vi "PSUSettingsMenu.vi"(0 "Enable":bool=TRUE, 5 "error in (no error)":errorcluster, 16 "PSU Calc":T1={"Low speed (km/s)"=2000.0, "High speed (km/s)"=3000.0, "Window (Delta-T)"=0.0, "Lower Cutoff"=0.0, "Multiplier"=0, "Low Charge (fC)"=2000.0, "High Charge (fC)"=2000.0, "High Mass (kg)"=2000.0, "Low Mass (kg)"=2000.0, "High Radius (µm) "=0.0, "Low Radius (µm)"=2000.0, "Exp. Voltage (MV)"=2000.0} {"Exp. Voltage (MV)" step=0.01 format="%#.6f"; "Window (Delta-T)" step=1.0 format="%#.0f"; "High Radius (µm)" min=0.0 max=1000.0; "High Mass (kg)" min=0.0 max=1.0; "High Charge (fC)" min=0.0 max=1000000000000.0; "High speed (km/s)" min=0.0 max=299790.0; "Low speed (km/s)" min=0.0 max=299790.0; "Low Charge (fC)" min=0.0 max=1000000000000.0; "Low Mass (kg)" min=0.0 max=1.0; "Low Radius (µm)" min=0.0 max=299792000.0; "Lower Cutoff" step=1.0 format="%#.0f"; "Multiplier" items=["1k", "10k"]}) -> (14 "Cancel 2":bool caption="Cancel", 18 "OK":bool, 19 "error out":errorcluster)   [LabVIEW 2012]
doc: "Displays a standard dialog box that prompts users to enter information, such as a user name and password.\n--------------------\n\nThis Express VI is configured as follows:\n\nMessage to Display to the User:Please Enter Experiment Settings Information For Database Storage.\nThe inputs are: \nNumber: Please Enter Group ID\nText Entry Box: Please Enter Tags:\nText Entry Box: Please Enter Experiment Description:"
uses:
  PSU Calc.ctl
  <vilib>/addons/database/Connection.llb/Conn Execute.vi
  <vilib>/addons/database/Recordset.llb/Rec Fetch Recordset Data (R).vi
  <vilib>/addons/database/Recordset.llb/Rec Destroy - Connection.vi
  PSU updated.vi
  <vilib>/addons/database/_DB Variant To Data/Database Variant To Data.xnode
  <vilib>/addons/database/NI_Database_API.lvlib
panel:
  out "Dust Density\n(kg/m^3)":dbl
  in  "Variable 2":enum32{"Velocity", "Charge", "Mass"}(radio)
  in  "Variable 1":enum32{"Velocity", "Charge", "Mass"}(radio)
  out "Lower Cutoff":dbl
  out "Window (Delta-T)":dbl
  in  "PSU update":bool caption="OK2"
  in  "Cancel":bool
  in  "OK1":bool
  # "Please Enter PSU Settings For Storage in the CCLDAS Database."
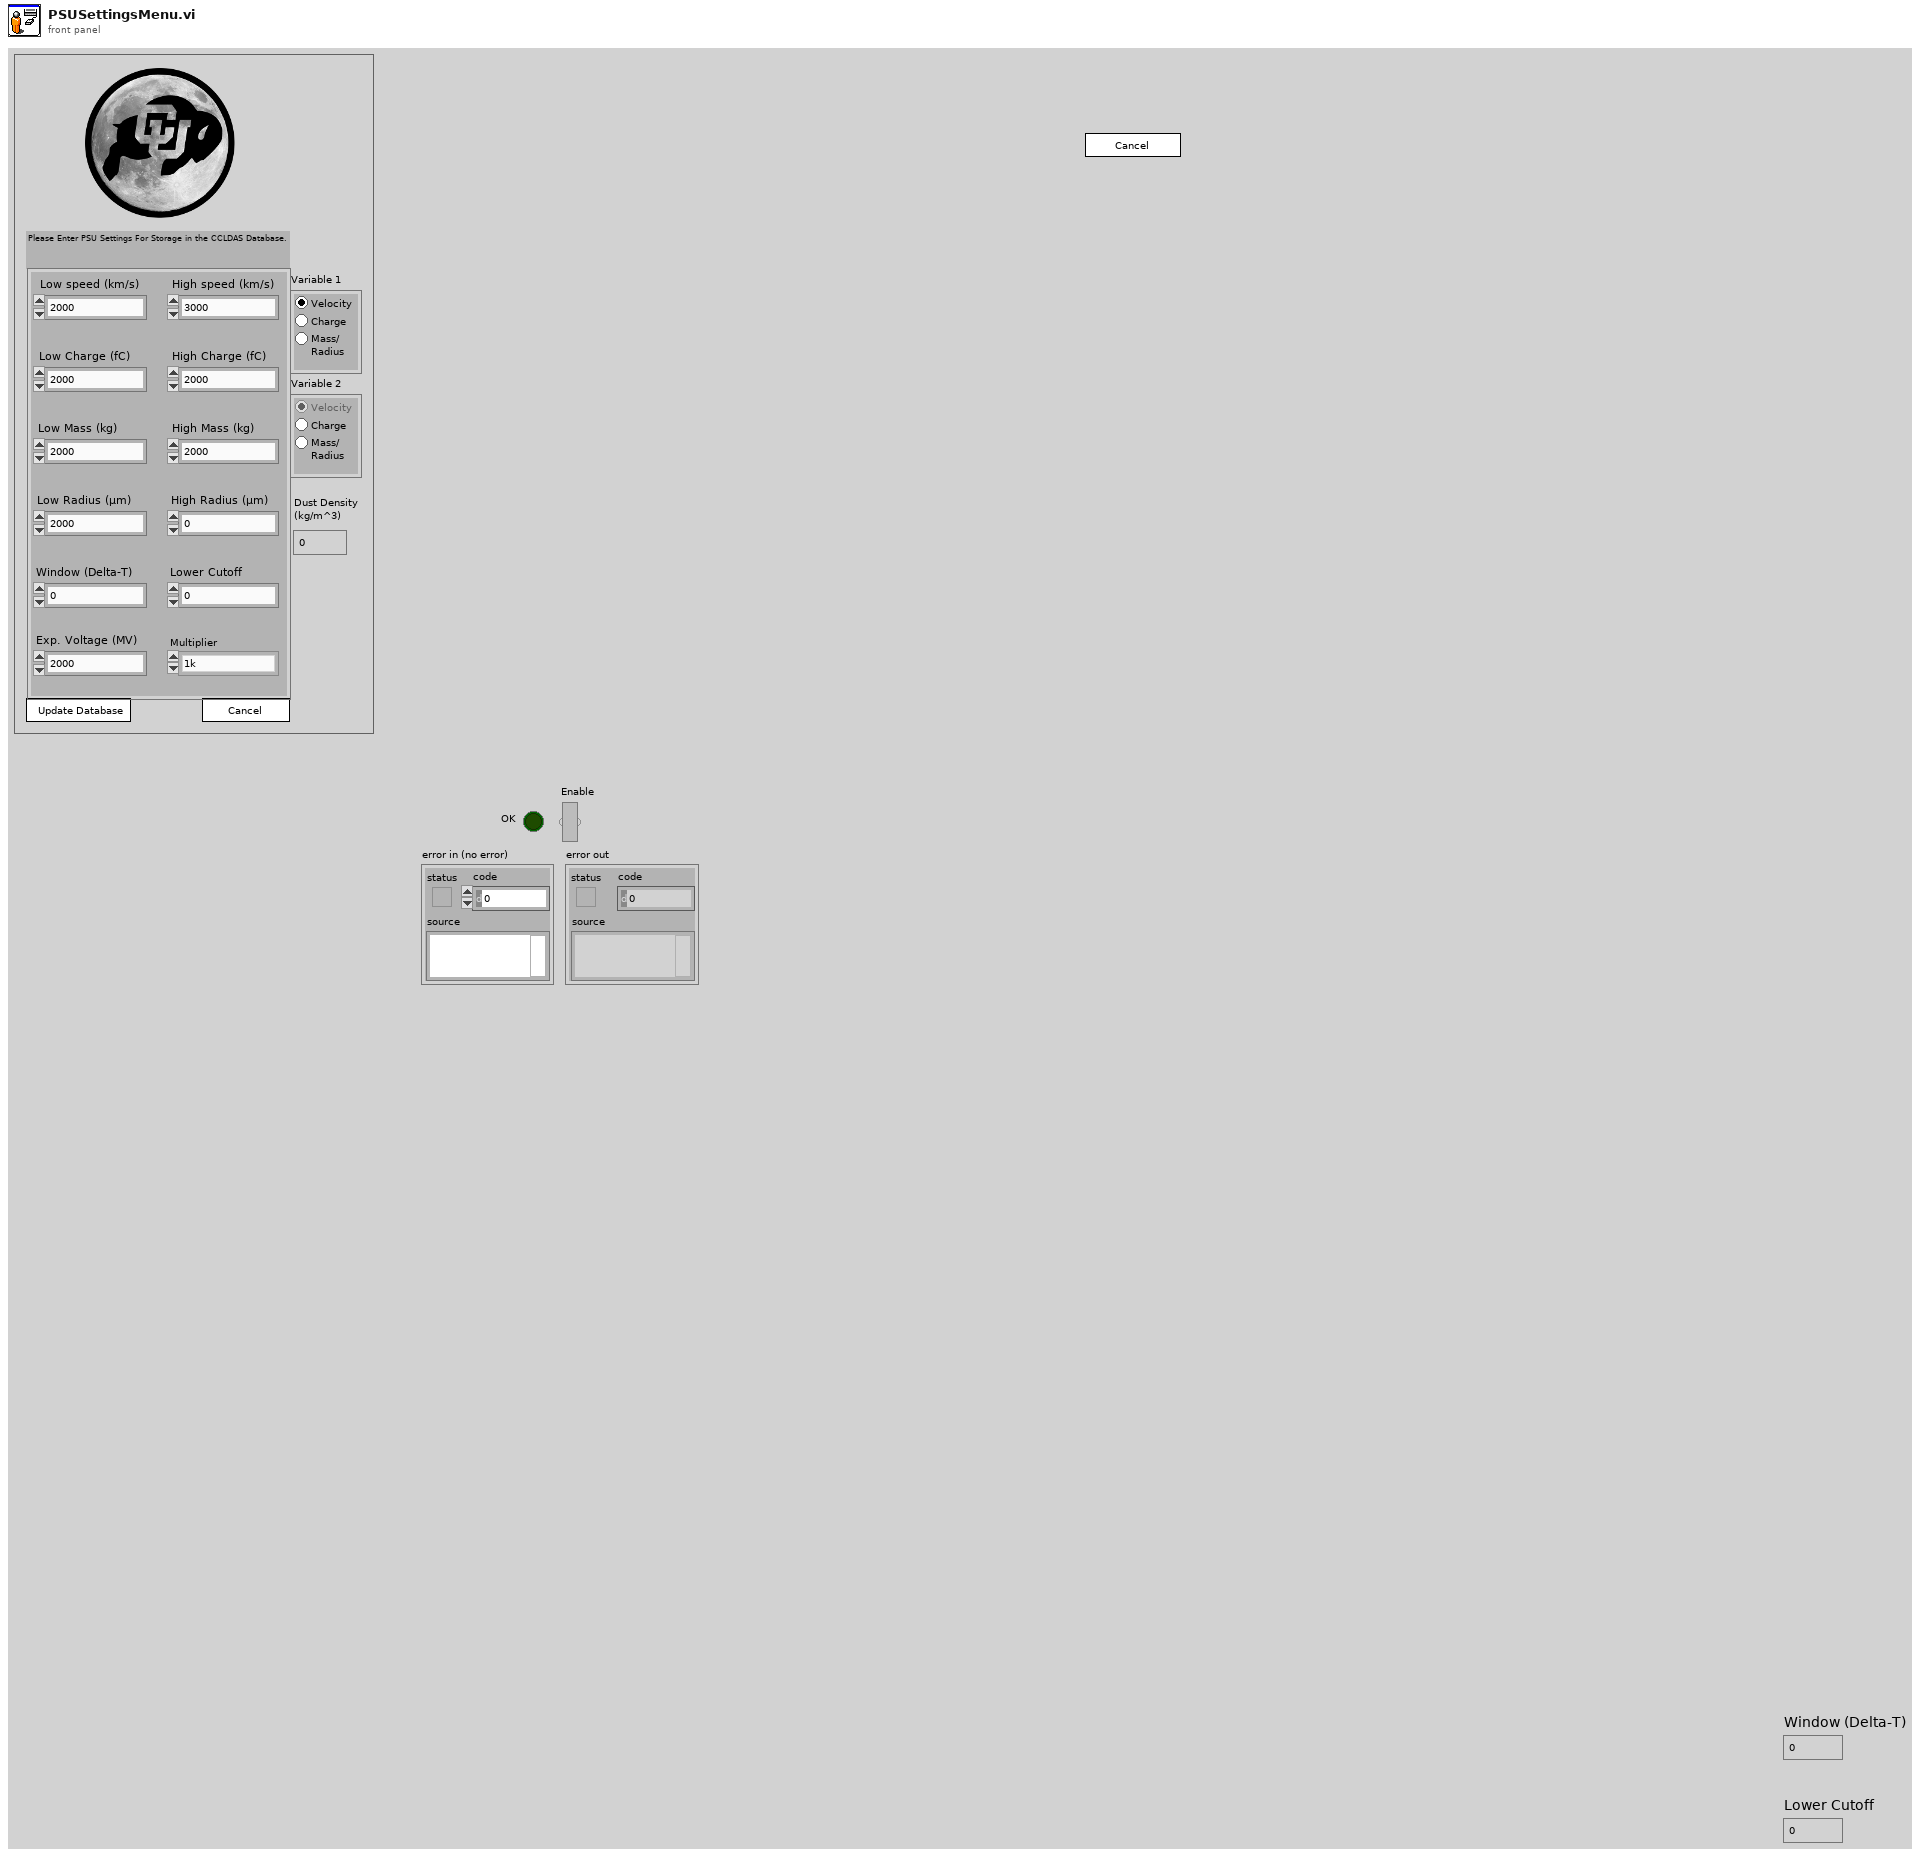
[diagram p1: front panel]
types:
  T1 = typedef "PSU Calc.ctl" = cluster{"Low speed (km/s)":dbl, "High speed (km/s)":dbl, "Window (Delta-T)":dbl, "Lower Cutoff":dbl, "Multiplier":u16, "Low Charge (fC)":dbl, "High Charge (fC)":dbl, "High Mass (kg)":dbl, "Low Mass (kg)":dbl, "High Radius (µm) ":dbl, "Low Radius (µm)":dbl, "Exp. Voltage (MV)":dbl}
  T2 = enum8{"Enabled", "Disabled", "Disabled and Grayed Out"}
  T3 = cluster{"Integer Timestamp":dbl, "Max Velocity":dbl, "Min Velocity":dbl, "Max Charge":dbl, "Min Charge":dbl, "Max Mass":dbl, "Min Mass":dbl, "Variable 1":enum8{"Velocity", "Charge", "Mass"}, "Variable 2":enum8{"Velocity", "Charge", "Mass"}}
  T4 = typedef "NI_Database_API.lvlib/Conn ObjectReference.ctl" = refnum<k1>
  T5 = typedef "NI_Database_API.lvlib/Rec ObjectReference.ctl" = refnum<k1>
  T6 = cluster{"Integer Timestamp":dbl, "Max Velocity":dbl, "Min Velocity":dbl, "Max Charge":dbl, "Min Charge":dbl, "Max Mass":dbl, "Min Mass":dbl, "Variable 1":enum32{"Velocity", "Charge", "Mass", "Radius"}, "Variable 2":enum32{"Velocity", "Charge", "Mass", "Radius"}}
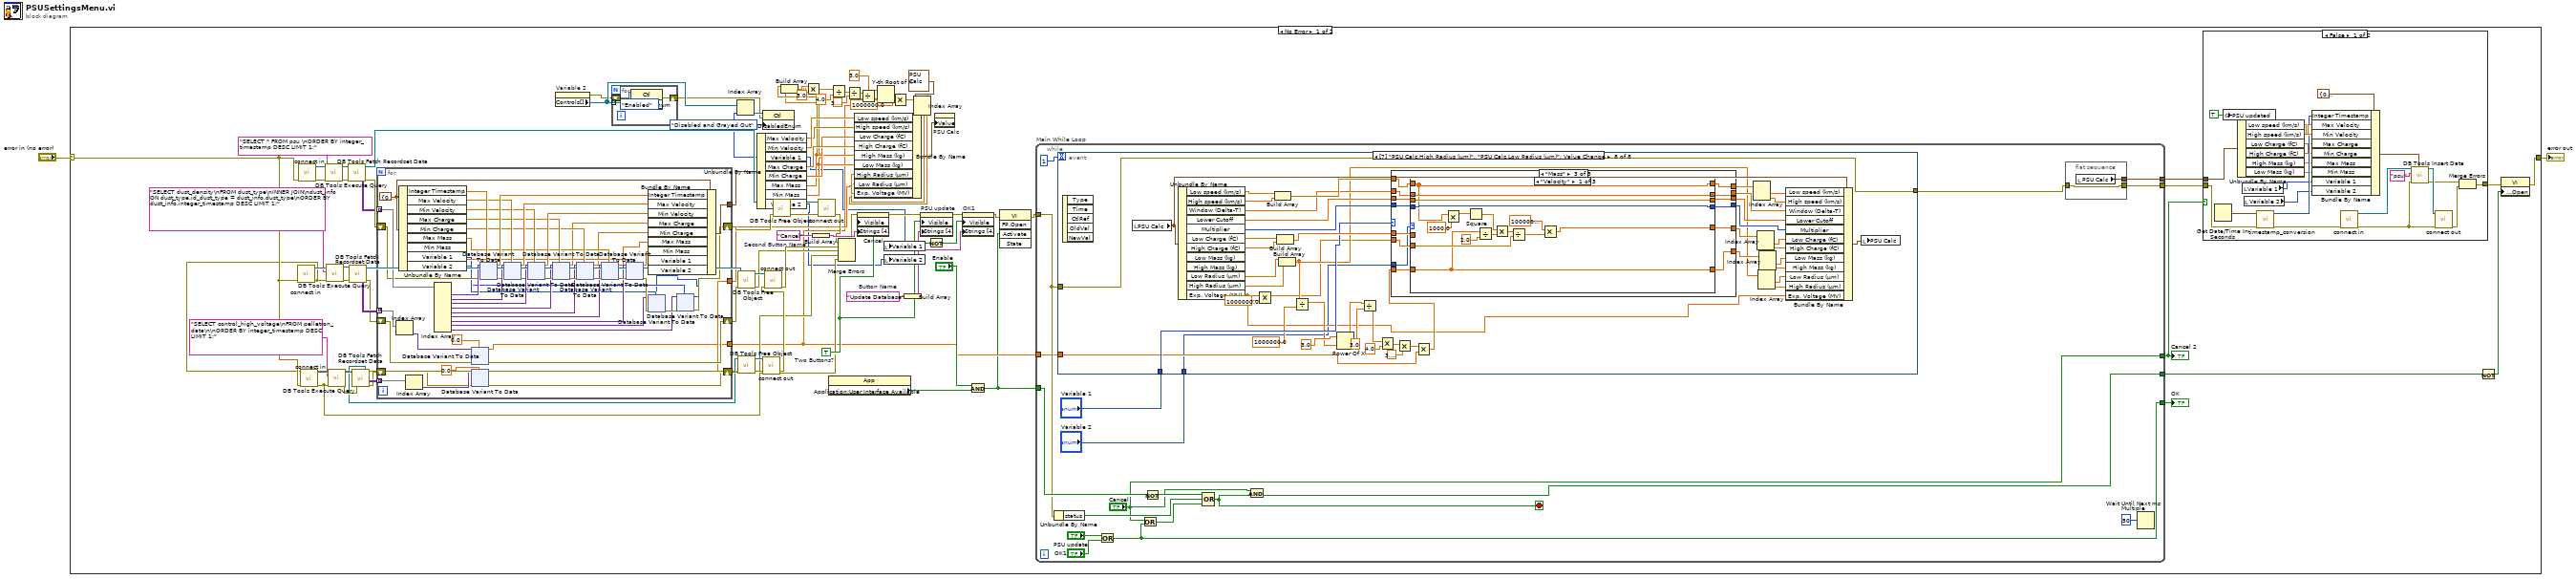
[diagram p0: block diagram]
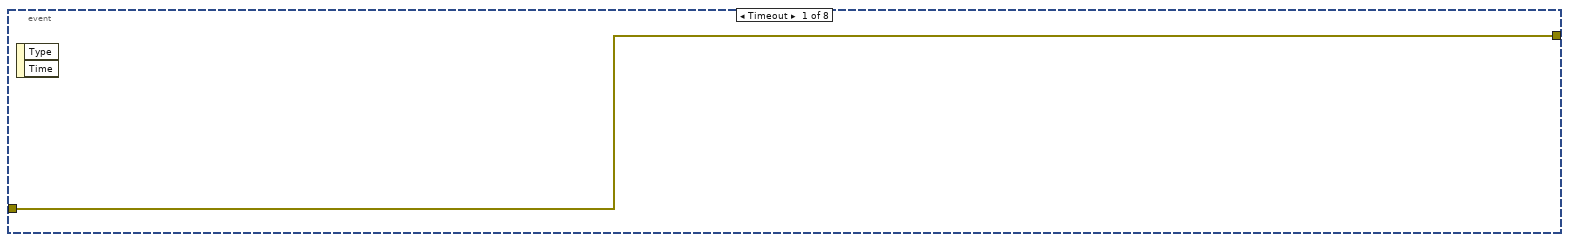
[diagram p3: hidden frame]
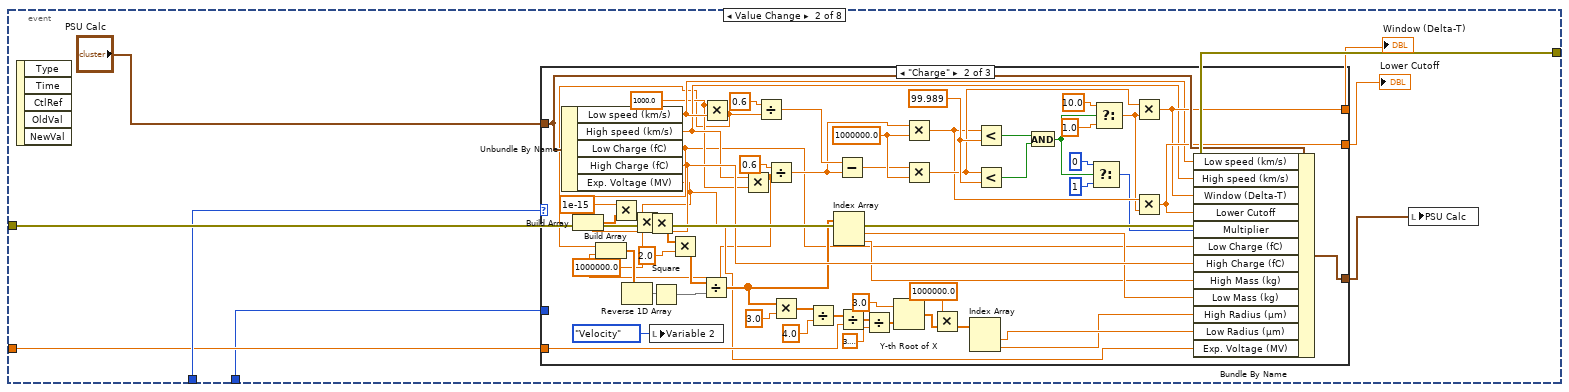
[diagram p4: hidden frame]
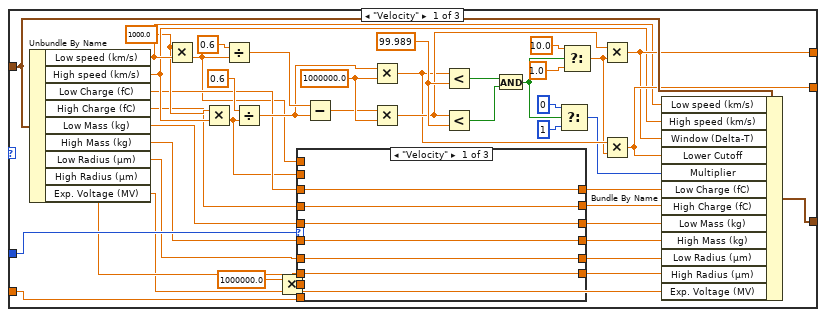
[diagram p5: hidden frame]
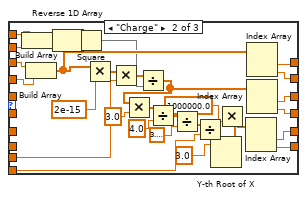
[diagram p6: hidden frame]
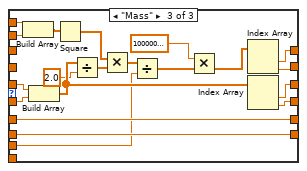
[diagram p7: hidden frame]
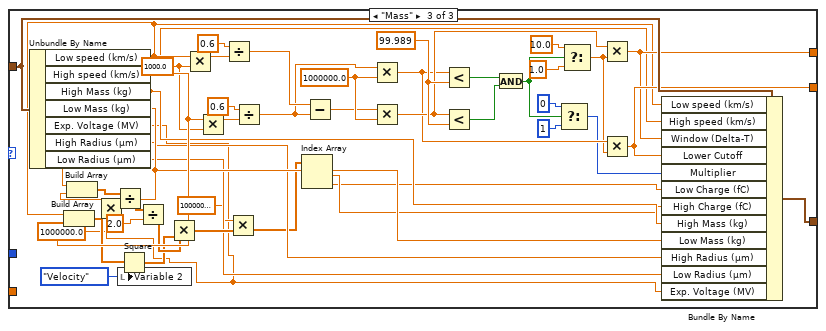
[diagram p8: hidden frame]
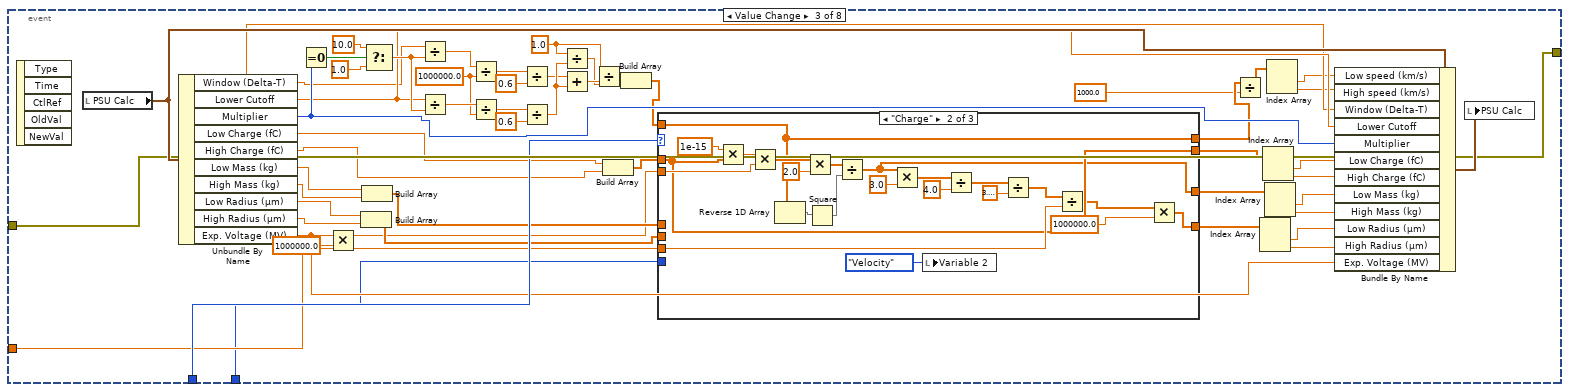
[diagram p9: hidden frame]
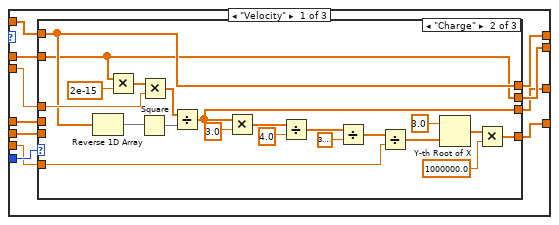
[diagram p10: hidden frame]
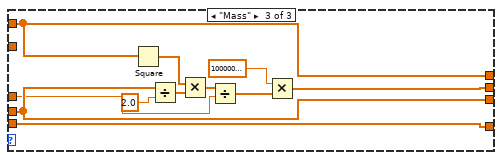
[diagram p12: hidden frame]
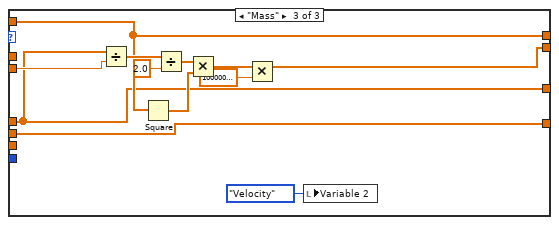
[diagram p13: hidden frame]
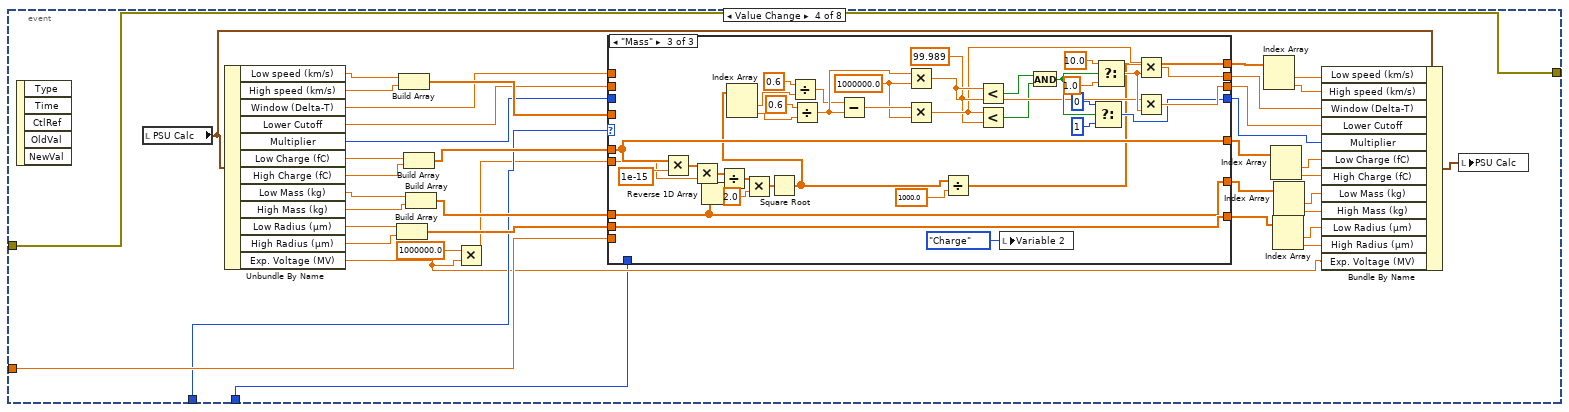
[diagram p14: hidden frame]
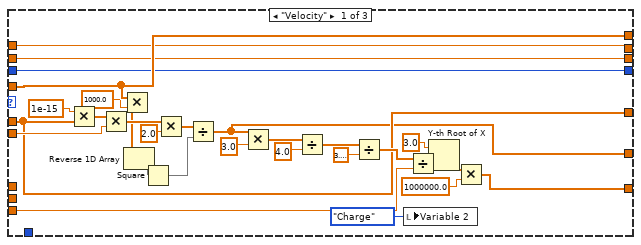
[diagram p15: hidden frame]
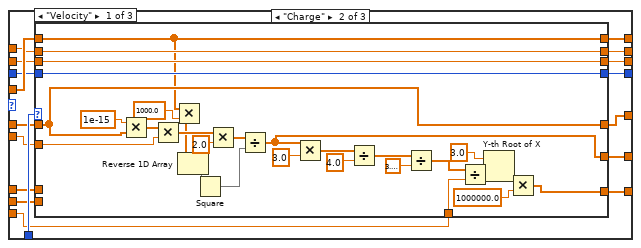
[diagram p16: hidden frame]
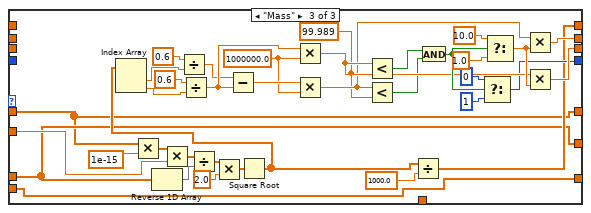
[diagram p18: hidden frame]
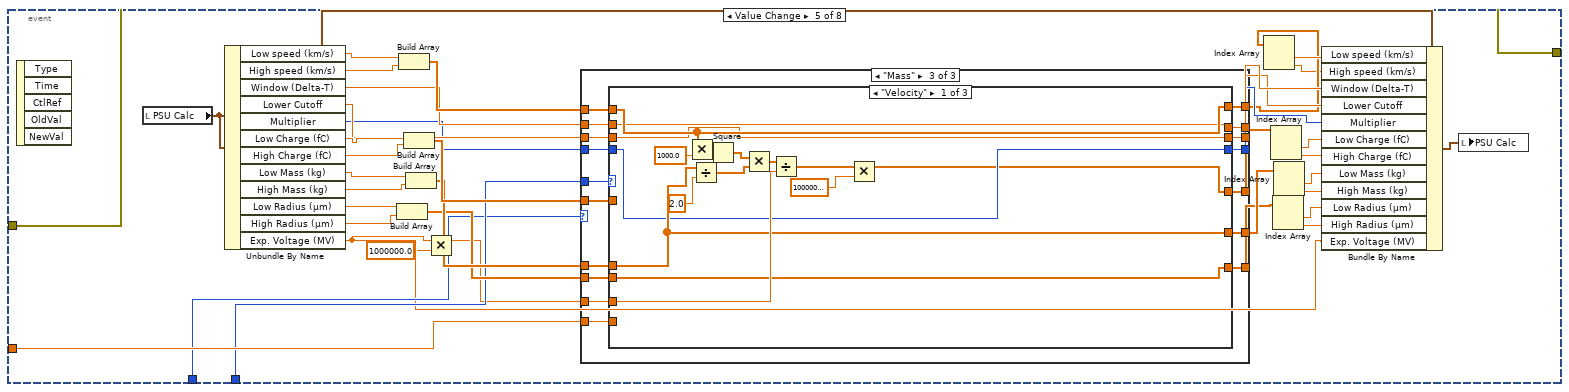
[diagram p19: hidden frame]
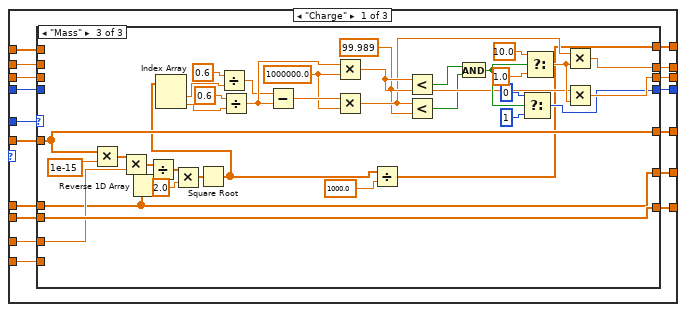
[diagram p20: hidden frame]
diagram:
  n1 = case shown="No Error" "error in (no error)" {
    selector: "error in (no error)" -> [w51 w1704]
    tunnel: [w68 w1704] -> w1
    frame No Error {
      w77 = "Cancel"  # Second Button Name
      w79 = "Update Database"  # Button Name
      w69 = TRUE  # Two Buttons?
      n2 = call "connect in.vi"("error in (no error)"=w51) -> ("error out"=w37:errorcluster, "Database Connection"=w57:T4)  [unwired: 6 in, 1 out]
      n3 = call "connect in.vi"("error in (no error)"=w51) -> ("error out"=w85:errorcluster, "Database Connection"=w84:T4)  [unwired: 6 in, 1 out]
      n4 = call "connect in.vi"("error in (no error)"=w51) -> ("error out"=w38:errorcluster, "Database Connection"=w50:T4)  [unwired: 6 in, 1 out]
      n5 = call-poly <vilib>:"DB Tools Execute Query.vi"("error in (no error)"=w85, "SQL query"="SELECT * FROM psu \nORDER BY integer_timestamp DESC LIMIT 1;", "connection reference"=w84) -> ("error out"=w87:errorcluster, "recordset reference"=w86:T5)  [unwired: 5 in]
      n6 = call-poly <vilib>:"DB Tools Execute Query.vi"("error in (no error)"=w37, "SQL query"="SELECT dust_density\nFROM dust_type\nINNER JOIN\ndust_info ON dust_type.id_dust_type = dust_info.dust_type\nORDER BY dust_info.integer_timestamp DESC LIMIT 1;", "connection reference"=w57) -> ("error out"=w54:errorcluster, "recordset reference"=w55:T5)  [unwired: 5 in]
      n7 = call-poly <vilib>:"DB Tools Execute Query.vi"("error in (no error)"=w38, "SQL query"="SELECT control_high_voltage\nFROM pelletron_data\n\nORDER BY integer_timestamp DESC LIMIT 1;", "connection reference"=w50) -> ("error out"=w49:errorcluster, "recordset reference"=w48:T5)  [unwired: 5 in]
      n8 = call-poly <vilib>:"DB Tools Fetch Recordset Data.vi"("error in (no error)"=w87, "recordset reference"=w86) -> ("error out"=w93:errorcluster, "recordset data"=w92:variant[][], "recordset reference out"=w88:T5)  [unwired: 3 in]
      n9 = call-poly <vilib>:"DB Tools Fetch Recordset Data.vi"("error in (no error)"=w54, "recordset reference"=w55) -> ("error out"=w52:errorcluster, "recordset data"=w53:variant[][], "recordset reference out"=w41:T5)  [unwired: 3 in]
      n10 = call-poly <vilib>:"DB Tools Fetch Recordset Data.vi"("error in (no error)"=w49, "recordset reference"=w48) -> ("error out"=w45:errorcluster, "recordset data"=w47:variant[][], "recordset reference out"=w42:T5)  [unwired: 3 in]
      n11 = for {
        tunnel: w92 -> [w173] mode=indexing
        shift-right: [w132] -> w62
        shift-left: w93 -> [w169]
        tunnel: [w168] -> w67
        tunnel: w53 -> [w142] mode=indexing
        shift-right: [w136] -> w44
        shift-left: w52 -> [w137]
        tunnel: w47 -> [w141] mode=indexing
        shift-right: [w135] -> w43
        shift-left: w45 -> [w138]
        tunnel: [w124] -> w26
        tunnel: [w122] -> w16
        w163 = T6 {"Integer Timestamp"=0.0, "Max Velocity"=0.0, "Min Velocity"=0.0, "Max Charge"=0.0, "Min Charge"=0.0, "Max Mass"=0.0, "Min Mass"=0.0, "Variable 1"=enum."Velocity", "Variable 2"=enum."Velocity"} ("PSU settings")
        n12 = Index Array(array=w142) -> (element=w140:variant)  [unwired: 1 in]
        n13 = Unbundle By Name(w163) -> ("Integer Timestamp"=w167:dbl, "Max Velocity"=w164:dbl, "Min Velocity"=w161:dbl, "Max Charge"=w150:dbl, "Min Charge"=w149:dbl, "Max Mass"=w148:dbl, "Min Mass"=w147:dbl, "Variable 1"=w129:enum32{"Velocity", "Charge", "Mass", "Radius"}, "Variable 2"=w128:enum32{"Velocity", "Charge", "Mass", "Radius"})
        n14 = Index Array(array=w141) -> (element=w139:variant)  [unwired: 1 in]
        n15 = Index Array(array=w173) -> (element #1=w172:variant, element #2=w171:variant, element #3=w162:variant, element #4=w155:variant, element #5=w154:variant, element #6=w153:variant, element #7=w151:variant, element #8=w131:variant, element #9=w130:variant)  [unwired: 9 in]
        n16 = xnode "Database Variant To Data"("database variant"=w140, "error in (no error)"=w137, "type"=0.0) -> ("data"=w122:dbl, "error out"=w136:errorcluster)
        n17 = xnode "Database Variant To Data"("database variant"=w139, "error in (no error)"=w138, "type"=0.0) -> ("data"=w124:dbl, "error out"=w135:errorcluster)
        n18 = xnode "Database Variant To Data"("database variant"=w172, "error in"=w169, "type"=w167) -> ("data"=w166:dbl, "error out"=w170:errorcluster)
        n19 = xnode "Database Variant To Data"("database variant"=w171, "error in"=w170, "type"=w164) -> ("data"=w165:dbl, "error out"=w159:errorcluster)
        n20 = xnode "Database Variant To Data"("database variant"=w162, "error in"=w159, "type"=w161) -> ("data"=w160:dbl, "error out"=w156:errorcluster)
        n21 = xnode "Database Variant To Data"("database variant"=w155, "error in (no error)"=w156, "type"=w150) -> ("data"=w146:dbl, "error out"=w158:errorcluster)
        n22 = xnode "Database Variant To Data"("database variant"=w154, "error in (no error)"=w158, "type"=w149) -> ("data"=w145:dbl, "error out"=w157:errorcluster)
        n23 = xnode "Database Variant To Data"("database variant"=w153, "error in (no error)"=w157, "type"=w148) -> ("data"=w144:dbl, "error out"=w152:errorcluster)
        n24 = xnode "Database Variant To Data"("database variant"=w151, "error in (no error)"=w152, "type"=w147) -> ("data"=w143:dbl, "error out"=w133:errorcluster)
        n25 = xnode "Database Variant To Data"("database variant"=w131, "error in (no error)"=w133, "type"=w129) -> ("data"=w127:enum32{"Velocity", "Charge", "Mass", "Radius"}, "error out"=w134:errorcluster)
        n26 = xnode "Database Variant To Data"("database variant"=w130, "error in (no error)"=w134, "type"=w128) -> ("data"=w126:enum32{"Velocity", "Charge", "Mass", "Radius"}, "error out"=w132:errorcluster)
        n27 = Bundle By Name(cluster=w163, "Integer Timestamp"=w166, "Max Velocity"=w165, "Min Velocity"=w160, "Max Charge"=w146, "Min Charge"=w145, "Max Mass"=w144, "Min Mass"=w143, "Variable 1"=w127, "Variable 2"=w126) -> (w168:T6)
      }
      n28 = property on="Variable 2" class="RadioBtnsControl (strict)"() -> (error out=w7:errorcluster, "Controls[]"=w8:refnum<vi>[])  [unwired: 2 in, 1 out]
      n29 = for {
        tunnel: w8 -> [w97] mode=indexing
        shift-right: [w94] -> w6
        shift-left: w7 -> [w96]
        n30 = property class="Ctl"(reference=w97, error in=w96, "DisabledEnum"=T2."Enabled" ("Disabled")) -> (error out=w94:errorcluster)  [unwired: 1 out]
      }
      n31 = call-poly <vilib>:"DB Tools Free Object.vi"("error in (no error)"=w44, "recordset reference"=w41) -> ("error out"=w35:errorcluster, "connection reference"=w40:T4)  [unwired: 8 in]
      n32 = call-poly <vilib>:"DB Tools Free Object.vi"("error in (no error)"=w43, "recordset reference"=w42) -> ("error out"=w33:errorcluster, "connection reference"=w39:T4)  [unwired: 8 in]
      n33 = Unbundle By Name(w67) -> ("Max Velocity"=w63:dbl, "Min Velocity"=w64:dbl, "Variable 1"=w5:enum32{"Velocity", "Charge", "Mass", "Radius"}, "Max Charge"=w28:dbl, "Min Charge"=w27:dbl, "Max Mass"=w25:dbl, "Min Mass"=w24:dbl, "Variable 2"=w4:enum32{"Velocity", "Charge", "Mass", "Radius"})
      n34 = Index Array(array=w8, index=w5) -> (element=w30:refnum<vi>)
      n35 = property class="Ctl"(reference=w30, error in=w6, "DisabledEnum"=T2."Disabled and Grayed Out" ("Disabled")) -> ()  [unwired: 2 out]
      n36 = call "connect out.vi"("error in (no error)"=w38, "connection reference"=w39) -> ("error out"=w34:errorcluster)  [unwired: 9 in]
      n37 = call "connect out.vi"("error in (no error)"=w37, "connection reference"=w40) -> ("error out"=w36:errorcluster)  [unwired: 9 in]
      n38 = call-poly <vilib>:"DB Tools Free Object.vi"("error in (no error)"=w62, "recordset reference"=w88) -> ("error out"=w89:errorcluster, "connection reference"=w90:T4)  [unwired: 8 in]
      n39 = Build Array(w25, w24) -> (w23:dbl[])
      n40 = Multiply(x=w23, y=3.0 ("Min Mass")) -> (x*y=w21:dbl[])
      n41 = Build Array(w77) -> (w76:string[])
      n42 = call "connect out.vi"("error in (no error)"=w89, "connection reference"=w90) -> ("error out"=w32:errorcluster)  [unwired: 9 in]
      n43 = property class="App"() -> ("Application:User Interface Available"=w82:bool)  [unwired: 2 in, 2 out]
      n44 = Divide(x=w21, y=4.0 ("Min Mass")) -> (x/y=w19:dbl[])
      n45 = Merge Errors(w32, w36, w35, w33, w34) -> (w31:errorcluster)
      n46 = Divide(x=w19, y=3.141592653589793) -> (x/y=w17:dbl[])
      n47 = property on="Cancel" class="Bool"(error in=w31, "Visible"=w69, "Strings [4]"=w76) -> (error out=w72:errorcluster)  [unwired: 1 in, 1 out]
      n48 = Divide(x=w17, y=w16) -> (x/y=w15:dbl[])
      n49 = Y-th Root of X(1:w15, 2:3.0 ("Min Mass")) -> (0:w11:dbl[])
      n50 = local write "Variable 1"(w5) -> ()
      n51 = local write "Variable 2"(w4) -> ()
      n52 = Multiply(x=w11, y=1000000.0 ("Min Mass")) -> (x*y=w10:dbl[])
      n53 = Build Array(w79) -> (w78:string[])
      n54 = Index Array(array=w10) -> (element #1=w14:dbl, element #2=w13:dbl)  [unwired: 2 in]
      n55 = Bundle By Name(cluster=T1 {"Low speed (km/s)"=2000.0, "High speed (km/s)"=3000.0, "Window (Delta-T)"=0.0, "Lower Cutoff"=0.0, "Multiplier"=0, "Low Charge (fC)"=0.0, "High Charge (fC)"=0.0, "High Mass (kg)"=0.0, "Low Mass (kg)"=0.0, "High Radius (µm) "=0.0, "Low Radius (µm)"=0.0, "Exp. Voltage (MV)"=0.0} ("PSU Calc"), "Low speed (km/s)"=w64, "High speed (km/s)"=w63, "Low Charge (fC)"=w27, "High Charge (fC)"=w28, "High Mass (kg)"=w25, "Low Mass (kg)"=w24, "High Radius (µm)"=w14, "Low Radius (µm)"=w13, "Exp. Voltage (MV)"=w26) -> (w66:T1)
      n56 = property on="PSU update" class="Bool"(error in=w72, "Visible"=w69, "Strings [4]"=w78) -> (error out=w73:errorcluster)  [unwired: 1 in, 1 out]
      n57 = Not(x=w69) -> (.not. x?=w71:bool)
      n58 = property on="PSU Calc" class="Clust (strict)"("Value"=w66) -> ()  [unwired: 2 in, 2 out]
      n59 = property on="OK1" class="Bool"(error in=w73, "Visible"=w71, "Strings [4]"=w78) -> (error out=w80:errorcluster)  [unwired: 1 in, 1 out]
      n60 = And(x="Enable", y=w82) -> (x .and. y?=w3:bool)
      n61 = invoke class="VI" method="FP.Open"(error in=w80, "Activate"=w3) -> (error out=w83:errorcluster)  [unwired: 3 in, 4 out]
      n62 = while "Main While Loop" {
        tunnel: [w541] -> w70
        tunnel: w3 -> [w539]
        tunnel: [w535] -> w75
        tunnel: w83 -> [w533]
        tunnel: [w531] -> w60
        tunnel: ["Cancel"] -> w61
        tunnel: [w529] -> w58
        tunnel: w16 -> [w527]
        stop <- w535 stop-if-true
        n63 = Unbundle By Name(w533) -> ("status"=w536:bool)
        n64 = event shown="[7] \"PSU Calc.High Radius (µm)\", \"PSU Calc.Low Radius (µm)\": Value Change" {
          selector: _ -> [_ _ _ _ _ _ _ _]
          dyn-events: _ -> [_ _ _ _ _ _ _ _]
          timeout: 1 -> [_ _ _ _ _ _ _ _]
          tunnel: w533 -> [w546 w553 w811 w899 w1091 w1363 w1374 w1542]
          tunnel: [w546 w553 w811 w899 w1091 w1355 w1374 w1542] -> w530
          tunnel: "Variable 1" -> [_ w549 w792 w900 w1092 _ w1388 w1558]
          tunnel: w527 -> [_ w548 w785 w919 w1112 _ w1380 w1551]
          tunnel: "Variable 2" -> [_ w547 w761 w895 w1093 w1359 w1370 w1538]
          event Timeout {
            n65 = event-data() -> ()  [unwired: 1 in, 2 out]
          }
          event Value Change {
            n66 = event-data() -> ()  [unwired: 1 in, 5 out]
            n67 = case shown="\"Charge\"" w549 {
              tunnel: [w598 w714 w760] -> w554
              tunnel: "PSU Calc" -> [w597 w713 w759]
              tunnel: [w596 w712 w758] -> w551
              tunnel: [w595 w711 w757] -> w550
              tunnel: w548 -> [w557 w675 _]
              tunnel: w547 -> [w573 _ _]
              frame "Velocity" {
                w574 = 1000.0 ("x")
                w588 = 99.989
                w590 = 1000000.0 ("y")
                n68 = Unbundle By Name(w597) -> ("Low speed (km/s)"=w579:dbl, "High speed (km/s)"=w575:dbl, "Low Charge (fC)"=w572:dbl, "High Charge (fC)"=w570:dbl, "Low Mass (kg)"=w568:dbl, "High Mass (kg)"=w567:dbl, "Low Radius (µm)"=w564:dbl, "High Radius (µm)"=w562:dbl, "Exp. Voltage (MV)"=w560:dbl)
                n69 = Multiply(x=w574, y=w579) -> (x*y=w558:dbl)
                n70 = Multiply(x=w574, y=w575) -> (x*y=w559:dbl)
                n71 = Divide(x=0.6, y=w558) -> (x/y=w592:dbl)
                n72 = Divide(x=0.6, y=w559) -> (x/y=w591:dbl)
                n73 = Multiply(x=1000000.0, y=w560) -> (x*y=w556:dbl)
                n74 = case shown="\"Velocity\"" w573 {
                  tunnel: w572 -> [w604 w632 _]
                  tunnel: [w604 w631 w649] -> w571
                  tunnel: w570 -> [w603 w633 _]
                  tunnel: [w603 w626 w646] -> w569
                  tunnel: w568 -> [w602 _ w653]
                  tunnel: [w602 w630 w648] -> w566
                  tunnel: w567 -> [w601 _ w652]
                  tunnel: [w601 w629 w647] -> w565
                  tunnel: w564 -> [w600 _ w651]
                  tunnel: [w600 w628 w651] -> w563
                  tunnel: w562 -> [w599 _ w650]
                  tunnel: [w599 w627 w650] -> w561
                  tunnel: w556 -> [_ w622 w639]
                  tunnel: w559 -> [_ w634 w654]
                  tunnel: w558 -> [_ w635 w655]
                  tunnel: w557 -> [_ w609 _]
                  frame "Velocity" {
                  }
                  frame "Charge" {
                    n75 = Build Array(w635, w634) -> (w620:dbl[])
                    n76 = Build Array(w632, w633) -> (w625:dbl[])
                    n77 = Reverse 1D Array(array=w620) -> (reversed array=w605:dbl[])
                    n78 = Square(x=w605) -> (x^2=w619:dbl[])
                    n79 = Multiply(x=w625, y=2e-15 ("x")) -> (x*y=w623:dbl[])
                    n80 = Multiply(x=w623, y=w622) -> (x*y=w621:dbl[])
                    n81 = Divide(x=w621, y=w619) -> (x/y=w618:dbl[])
                    n82 = Multiply(x=w618, y=3.0 ("x")) -> (x*y=w616:dbl[])
                    n83 = Divide(x=w616, y=4.0 ("x")) -> (x/y=w615:dbl[])
                    n84 = Divide(x=w615, y=3.141592653589793) -> (x/y=w614:dbl[])
                    n85 = Divide(x=w614, y=w609) -> (x/y=w613:dbl[])
                    n86 = Y-th Root of X(1:w613, 2:3.0 ("x")) -> (0:w608:dbl[])
                    n87 = Multiply(x=w608, y=1000000.0 ("x")) -> (x*y=w607:dbl[])
                    n88 = Index Array(array=w607) -> (element #1=w628:dbl, element #2=w627:dbl)  [unwired: 2 in]
                    n89 = Index Array(array=w625) -> (element #1=w631:dbl, element #2=w626:dbl)  [unwired: 2 in]
                    n90 = Index Array(array=w618) -> (element #1=w630:dbl, element #2=w629:dbl)  [unwired: 2 in]
                  }
                  frame "Mass" {
                    n91 = Build Array(w655, w654) -> (w645:dbl[])
                    n92 = Build Array(w653, w652) -> (w644:dbl[])
                    n93 = Square(x=w645) -> (x^2=w641:dbl[])
                    n94 = Divide(x=w644, y=2.0 ("x")) -> (x/y=w642:dbl[])
                    n95 = Multiply(x=w641, y=w642) -> (x*y=w640:dbl[])
                    n96 = Divide(x=w640, y=w639) -> (x/y=w638:dbl[])
                    n97 = Multiply(x=1000000000000000.0, y=w638) -> (x*y=w637:dbl[])
                    n98 = Index Array(array=w637) -> (element #1=w649:dbl, element #2=w646:dbl)  [unwired: 2 in]
                    n99 = Index Array(array=w644) -> (element #1=w648:dbl, element #2=w647:dbl)  [unwired: 2 in]
                  }
                }
                n100 = Subtract(x=w592, y=w591) -> (x-y=w589:dbl)
                n101 = Multiply(x=w591, y=w590) -> (x*y=w582:dbl)
                n102 = Multiply(x=w589, y=w590) -> (x*y=w583:dbl)
                n103 = Less?(x=w582, y=w588) -> (x < y?=w587:bool)
                n104 = Less?(x=w583, y=w588) -> (x < y?=w586:bool)
                n105 = And(x=w587, y=w586) -> (x .and. y?=w580:bool)
                n106 = Select(t=u16 0 ("Multiplier"), s=w580, f=u16 1 ("Multiplier")) -> (s? t:f=w576:u16)
                n107 = Select(t=10.0, s=w580, f=1.0) -> (s? t:f=w581:dbl)
                n108 = Multiply(x=w583, y=w581) -> (x*y=w595:dbl)
                n109 = Multiply(x=w582, y=w581) -> (x*y=w596:dbl)
                n110 = Bundle By Name(cluster=w597, "Low speed (km/s)"=w579, "High speed (km/s)"=w575, "Window (Delta-T)"=w595, "Lower Cutoff"=w596, "Multiplier"=w576, "Low Charge (fC)"=w571, "High Charge (fC)"=w569, "Low Mass (kg)"=w566, "High Mass (kg)"=w565, "Low Radius (µm)"=w563, "High Radius (µm)"=w561, "Exp. Voltage (MV)"=w560) -> (w598:T1)
              }
              frame "Charge" {
                w663 = 1000.0 ("x")
                w704 = 99.989
                w706 = 1000000.0 ("y")
                n111 = Unbundle By Name(w713) -> ("Low speed (km/s)"=w687:dbl, "High speed (km/s)"=w686:dbl, "Low Charge (fC)"=w662:dbl, "High Charge (fC)"=w691:dbl, "Exp. Voltage (MV)"=w661:dbl)
                n112 = Build Array(w662, w691) -> (w690:dbl[])
                n113 = Multiply(x=1e-15, y=w690) -> (x*y=w667:dbl[])
                n114 = Multiply(x=w661, y=1000000.0) -> (x*y=w660:dbl)
                n115 = Multiply(x=w667, y=w660) -> (x*y=w689:dbl[])
                n116 = local write "Variable 2"(enum32{"Velocity", "Charge", "Mass"}."Velocity" ("Variable 2")) -> ()
                n117 = Multiply(x=w689, y=2.0) -> (x*y=w684:dbl[])
                n118 = Multiply(x=w663, y=w687) -> (x*y=w658:dbl)
                n119 = Multiply(x=w686, y=w663) -> (x*y=w657:dbl)
                n120 = Build Array(w658, w657) -> (w685:dbl[])
                n121 = Reverse 1D Array(array=w685) -> (reversed array=w656:dbl[])
                n122 = Square(x=w656) -> (x^2=w683:dbl[])
                n123 = Divide(x=w684, y=w683) -> (x/y=w680:dbl[])
                n124 = Divide(x=0.6, y=w658) -> (x/y=w708:dbl)
                n125 = Divide(x=0.6, y=w657) -> (x/y=w707:dbl)
                n126 = Multiply(x=w680, y=3.0) -> (x*y=w678:dbl[])
                n127 = Divide(x=w678, y=4.0) -> (x/y=w676:dbl[])
                n128 = Index Array(array=w680) -> (element #1=w682:dbl, element #2=w681:dbl)  [unwired: 2 in]
                n129 = Subtract(x=w708, y=w707) -> (x-y=w705:dbl)
                n130 = Divide(x=w676, y=w675) -> (x/y=w674:dbl[])
                n131 = Divide(x=w674, y=3.141592653589793) -> (x/y=w672:dbl[])
                n132 = Y-th Root of X(1:w672, 2:3.0) -> (0:w670:dbl[])
                n133 = Multiply(x=w707, y=w706) -> (x*y=w698:dbl)
                n134 = Multiply(x=w705, y=w706) -> (x*y=w699:dbl)
                n135 = Multiply(x=1000000.0, y=w670) -> (x*y=w665:dbl[])
                n136 = Index Array(array=w665) -> (element #1=w669:dbl, element #2=w668:dbl)  [unwired: 2 in]
                n137 = Less?(x=w698, y=w704) -> (x < y?=w703:bool)
                n138 = Less?(x=w699, y=w704) -> (x < y?=w702:bool)
                n139 = And(x=w703, y=w702) -> (x .and. y?=w696:bool)
                n140 = Select(t=u16 0 ("Multiplier"), s=w696, f=u16 1 ("Multiplier")) -> (s? t:f=w693:u16)
                n141 = Select(t=10.0, s=w696, f=1.0) -> (s? t:f=w697:dbl)
                n142 = Multiply(x=w699, y=w697) -> (x*y=w711:dbl)
                n143 = Multiply(x=w698, y=w697) -> (x*y=w712:dbl)
                n144 = Bundle By Name(cluster=w713, "Low speed (km/s)"=w687, "High speed (km/s)"=w686, "Window (Delta-T)"=w711, "Lower Cutoff"=w712, "Multiplier"=w693, "Low Charge (fC)"=w662, "High Charge (fC)"=w691, "High Mass (kg)"=w681, "Low Mass (kg)"=w682, "High Radius (µm)"=w668, "Low Radius (µm)"=w669, "Exp. Voltage (MV)"=w661) -> (w714:T1)
              }
              frame "Mass" {
                w718 = 1000.0 ("y")
                w750 = 99.989
                w752 = 1000000.0 ("y")
                n145 = Unbundle By Name(w759) -> ("Low speed (km/s)"=w735:dbl, "High speed (km/s)"=w734:dbl, "High Mass (kg)"=w729:dbl, "Low Mass (kg)"=w728:dbl, "Exp. Voltage (MV)"=w717:dbl, "High Radius (µm)"=w724:dbl, "Low Radius (µm)"=w723:dbl)
                n146 = Build Array(w735, w734) -> (w733:dbl[])
                n147 = Build Array(w729, w728) -> (w725:dbl[])
                n148 = Multiply(x=w717, y=1000000.0) -> (x*y=w716:dbl)
                n149 = Divide(x=w725, y=w716) -> (x/y=w737:dbl[])
                n150 = local write "Variable 2"(enum32{"Velocity", "Charge", "Mass"}."Velocity" ("Variable 2")) -> ()
                n151 = Square(x=w733) -> (x^2=w731:dbl[])
                n152 = Divide(x=w737, y=2.0) -> (x/y=w732:dbl[])
                n153 = Multiply(x=w732, y=w731) -> (x*y=w730:dbl[])
                n154 = Multiply(x=w735, y=w718) -> (x*y=w720:dbl)
                n155 = Multiply(x=w734, y=w718) -> (x*y=w719:dbl)
                n156 = Divide(x=0.6, y=w720) -> (x/y=w754:dbl)
                n157 = Multiply(x=1000000000000000.0, y=w730) -> (x*y=w722:dbl[])
                n158 = Divide(x=0.6, y=w719) -> (x/y=w753:dbl)
                n159 = Index Array(array=w722) -> (element #1=w727:dbl, element #2=w726:dbl)  [unwired: 2 in]
                n160 = Subtract(x=w754, y=w753) -> (x-y=w751:dbl)
                n161 = Multiply(x=w753, y=w752) -> (x*y=w744:dbl)
                n162 = Multiply(x=w751, y=w752) -> (x*y=w745:dbl)
                n163 = Less?(x=w744, y=w750) -> (x < y?=w749:bool)
                n164 = Less?(x=w745, y=w750) -> (x < y?=w748:bool)
                n165 = And(x=w749, y=w748) -> (x .and. y?=w742:bool)
                n166 = Select(t=u16 0 ("Multiplier"), s=w742, f=u16 1 ("Multiplier")) -> (s? t:f=w739:u16)
                n167 = Select(t=10.0, s=w742, f=1.0) -> (s? t:f=w743:dbl)
                n168 = Multiply(x=w745, y=w743) -> (x*y=w757:dbl)
                n169 = Multiply(x=w744, y=w743) -> (x*y=w758:dbl)
                n170 = Bundle By Name(cluster=w759, "Low speed (km/s)"=w735, "High speed (km/s)"=w734, "Window (Delta-T)"=w757, "Lower Cutoff"=w758, "Multiplier"=w739, "Low Charge (fC)"=w726, "High Charge (fC)"=w727, "High Mass (kg)"=w729, "Low Mass (kg)"=w728, "High Radius (µm)"=w724, "Low Radius (µm)"=w723, "Exp. Voltage (MV)"=w717) -> (w760:T1)
              }
            }
            "Window (Delta-T)" <- w550
            "Lower Cutoff" <- w551
            n171 = local write "PSU Calc"(w554) -> ()
          }
          event Value Change {
            w804 = 1.0 ("x")
            w807 = 1000000.0 ("y")
            n172 = event-data() -> ()  [unwired: 1 in, 5 out]
            n173 = local read "PSU Calc"() -> (w813:T1)
            n174 = Unbundle By Name(w813) -> ("Window (Delta-T)"=w795:dbl, "Lower Cutoff"=w796:dbl, "Multiplier"=w798:u16, "Low Charge (fC)"=w788:dbl, "High Charge (fC)"=w787:dbl, "Low Mass (kg)"=w784:dbl, "High Mass (kg)"=w783:dbl, "Low Radius (µm)"=w782:dbl, "High Radius (µm)"=w781:dbl, "Exp. Voltage (MV)"=w764:dbl)
            n175 = Equal To 0?(x=w798) -> (x = 0?=w799:bool)
            n176 = Multiply(x=w764, y=1000000.0) -> (x*y=w763:dbl)
            n177 = Build Array(w782, w781) -> (w779:dbl[])
            n178 = Build Array(w784, w783) -> (w780:dbl[])
            n179 = Select(t=10.0, s=w799, f=1.0) -> (s? t:f=w797:dbl)
            n180 = Divide(x=w795, y=w797) -> (x/y=w810:dbl)
            n181 = Divide(x=w796, y=w797) -> (x/y=w808:dbl)
            n182 = Divide(x=w810, y=w807) -> (x/y=w802:dbl)
            n183 = Divide(x=w808, y=w807) -> (x/y=w805:dbl)
            n184 = Divide(x=w802, y=0.6) -> (x/y=w801:dbl)
            n185 = Divide(x=w805, y=0.6) -> (x/y=w803:dbl)
            n186 = Divide(x=w804, y=w803) -> (x/y=w790:dbl)
            n187 = Add(x=w801, y=w803) -> (x+y=w800:dbl)
            n188 = Divide(x=w804, y=w800) -> (x/y=w791:dbl)
            n189 = Build Array(w788, w787) -> (w786:dbl[])
            n190 = Build Array(w791, w790) -> (w789:dbl[])
            n191 = case shown="\"Charge\"" w792 {
              tunnel: w789 -> [w823 w870 w889]
              tunnel: w763 -> [w815 w876 w894]
              tunnel: w786 -> [w821 w869 _]
              tunnel: w785 -> [w814 w875 _]
              tunnel: w780 -> [w819 _ w887]
              tunnel: w779 -> [w817 _ w888]
              tunnel: [w822 w870 w889] -> w766
              tunnel: [w820 w869 w885] -> w776
              tunnel: [w818 w863 w887] -> w775
              tunnel: [w816 w865 w888] -> w774
              tunnel: w761 -> [w824 _ _]
              frame "Velocity" {
                n192 = case shown="\"Charge\"" w824 {
                  tunnel: w823 -> [w828 w832 w853]
                  tunnel: [w828 w832 w853] -> w822
                  tunnel: w821 -> [w827 w831 _]
                  tunnel: [w827 w831 w852] -> w820
                  tunnel: w819 -> [w826 _ w851]
                  tunnel: [w826 w833 w851] -> w818
                  tunnel: w817 -> [w825 _ w854]
                  tunnel: [w825 w830 w854] -> w816
                  tunnel: w815 -> [_ w835 w850]
                  tunnel: w814 -> [_ w834 _]
                  frame "Velocity" {
                  }
                  frame "Charge" {
                    n193 = Reverse 1D Array(array=w832) -> (reversed array=w829:dbl[])
                    n194 = Multiply(x=w831, y=2e-15 ("x")) -> (x*y=w837:dbl[])
                    n195 = Square(x=w829) -> (x^2=w839:dbl[])
                    n196 = Multiply(x=w837, y=w835) -> (x*y=w838:dbl[])
                    n197 = Divide(x=w838, y=w839) -> (x/y=w833:dbl[])
                    n198 = Multiply(x=w833, y=3.0 ("x")) -> (x*y=w841:dbl[])
                    n199 = Divide(x=w841, y=4.0 ("x")) -> (x/y=w842:dbl[])
                    n200 = Divide(x=w842, y=3.141592653589793) -> (x/y=w843:dbl[])
                    n201 = Divide(x=w843, y=w834) -> (x/y=w844:dbl[])
                    n202 = Y-th Root of X(1:w844, 2:3.0 ("x")) -> (0:w848:dbl[])
                    n203 = Multiply(x=w848, y=1000000.0 ("x")) -> (x*y=w830:dbl[])
                  }
                  frame "Mass" {
                    n204 = Square(x=w853) -> (x^2=w858:dbl[])
                    n205 = Divide(x=w851, y=2.0 ("x")) -> (x/y=w859:dbl[])
                    n206 = Multiply(x=w858, y=w859) -> (x*y=w857:dbl[])
                    n207 = Divide(x=w857, y=w850) -> (x/y=w856:dbl[])
                    n208 = Multiply(x=1000000000000000.0, y=w856) -> (x*y=w852:dbl[])
                  }
                }
              }
              frame "Charge" {
                n209 = Multiply(x=1e-15 ("Exp. Voltage (V)"), y=w869) -> (x*y=w867:dbl[])
                n210 = Multiply(x=w867, y=w876) -> (x*y=w874:dbl[])
                n211 = Reverse 1D Array(array=w870) -> (reversed array=w861:dbl[])
                n212 = Multiply(x=w874, y=2.0 ("Exp. Voltage (V)")) -> (x*y=w872:dbl[])
                n213 = Square(x=w861) -> (x^2=w871:dbl[])
                n214 = Divide(x=w872, y=w871) -> (x/y=w863:dbl[])
                n215 = Multiply(x=w863, y=3.0 ("Exp. Voltage (V)")) -> (x*y=w881:dbl[])
                n216 = local write "Variable 2"(enum32{"Velocity", "Charge", "Mass"}."Velocity" ("Variable 2")) -> ()
                n217 = Divide(x=w881, y=4.0 ("Exp. Voltage (V)")) -> (x/y=w879:dbl[])
                n218 = Divide(x=w879, y=3.141592653589793) -> (x/y=w877:dbl[])
                n219 = Divide(x=w877, y=w875) -> (x/y=w868:dbl[])
                n220 = Multiply(x=w868, y=1000000.0 ("Exp. Voltage (V)")) -> (x*y=w865:dbl[])
              }
              frame "Mass" {
                n221 = Divide(x=w887, y=w894) -> (x/y=w893:dbl[])
                n222 = Square(x=w889) -> (x^2=w890:dbl[])
                n223 = Divide(x=w893, y=2.0 ("Exp. Voltage (V)")) -> (x/y=w891:dbl[])
                n224 = Multiply(x=w891, y=w890) -> (x*y=w886:dbl[])
                n225 = Multiply(x=w886, y=1000000000000000.0 ("Exp. Voltage (V)")) -> (x*y=w885:dbl[])
                n226 = local write "Variable 2"(enum32{"Velocity", "Charge", "Mass"}."Velocity" ("Variable 2")) -> ()
              }
            }
            n227 = Divide(x=w766, y=1000.0 ("Exp. Voltage (V)")) -> (x/y=w767:dbl[])
            n228 = Index Array(array=w774) -> (element #1=w769:dbl, element #2=w768:dbl)  [unwired: 2 in]
            n229 = Index Array(array=w776) -> (element #1=w773:dbl, element #2=w772:dbl)  [unwired: 2 in]
            n230 = Index Array(array=w775) -> (element #1=w771:dbl, element #2=w770:dbl)  [unwired: 2 in]
            n231 = Index Array(array=w767) -> (element #1=w778:dbl, element #2=w777:dbl)  [unwired: 2 in]
            n232 = Bundle By Name(cluster=w813, "Low speed (km/s)"=w778, "High speed (km/s)"=w777, "Window (Delta-T)"=w795, "Lower Cutoff"=w796, "Multiplier"=w798, "Low Charge (fC)"=w773, "High Charge (fC)"=w772, "Low Mass (kg)"=w771, "High Mass (kg)"=w770, "Low Radius (µm)"=w769, "High Radius (µm)"=w768, "Exp. Voltage (MV)"=w764) -> (w812:T1)
            n233 = local write "PSU Calc"(w812) -> ()
          }
          event Value Change {
            n234 = event-data() -> ()  [unwired: 1 in, 5 out]
            n235 = local read "PSU Calc"() -> (w932:T1)
            n236 = Unbundle By Name(w932) -> ("Low speed (km/s)"=w931:dbl, "High speed (km/s)"=w930:dbl, "Window (Delta-T)"=w918:dbl, "Lower Cutoff"=w917:dbl, "Multiplier"=w916:u16, "Low Charge (fC)"=w928:dbl, "High Charge (fC)"=w927:dbl, "Low Mass (kg)"=w926:dbl, "High Mass (kg)"=w925:dbl, "Low Radius (µm)"=w924:dbl, "High Radius (µm)"=w923:dbl, "Exp. Voltage (MV)"=w898:dbl)
            n237 = Build Array(w924, w923) -> (w920:dbl[])
            n238 = Build Array(w931, w930) -> (w929:dbl[])
            n239 = Build Array(w928, w927) -> (w922:dbl[])
            n240 = Build Array(w926, w925) -> (w921:dbl[])
            n241 = Multiply(x=1000000.0, y=w898) -> (x*y=w897:dbl)
            n242 = case shown="\"Mass\"" w900 {
              tunnel: w929 -> [w943 w978 _]
              tunnel: w897 -> [w956 w964 w1061]
              tunnel: w922 -> [w950 w970 w1064]
              tunnel: w919 -> [w955 w963 _]
              tunnel: w921 -> [_ w968 w1059]
              tunnel: w920 -> [_ w966 w1087]
              tunnel: [w943 w977 w1054] -> w911
              tunnel: [w950 w969 w1064] -> w910
              tunnel: [w944 w967 w1059] -> w909
              tunnel: [w946 w965 w1087] -> w908
              tunnel: w918 -> [w942 w976 _]
              tunnel: w917 -> [w941 w974 _]
              tunnel: w916 -> [w940 w972 _]
              tunnel: [w942 w975 w1067] -> w915
              tunnel: [w941 w973 w1066] -> w914
              tunnel: [w940 w971 w1065] -> w913
              tunnel: w895 -> [_ w979 _]
              frame "Velocity" {
                n243 = Multiply(x=1e-15 ("Exp. Voltage (V)"), y=w950) -> (x*y=w948:dbl[])
                n244 = Multiply(x=w948, y=w956) -> (x*y=w954:dbl[])
                n245 = Multiply(x=w943, y=1000.0 ("Exp. Voltage (V)")) -> (x*y=w938:dbl[])
                n246 = Reverse 1D Array(array=w938) -> (reversed array=w934:dbl[])
                n247 = Square(x=w934) -> (x^2=w951:dbl[])
                n248 = Multiply(x=w954, y=2.0 ("Exp. Voltage (V)")) -> (x*y=w952:dbl[])
                n249 = Divide(x=w952, y=w951) -> (x/y=w944:dbl[])
                n250 = Multiply(x=w944, y=3.0 ("Exp. Voltage (V)")) -> (x*y=w961:dbl[])
                n251 = Divide(x=w961, y=4.0 ("Exp. Voltage (V)")) -> (x/y=w959:dbl[])
                n252 = Divide(x=w959, y=3.141592653589793) -> (x/y=w957:dbl[])
                n253 = local write "Variable 2"(enum32{"Velocity", "Charge", "Mass"}."Charge" ("Variable 2")) -> ()
                n254 = Divide(x=w957, y=w955) -> (x/y=w949:dbl[])
                n255 = Y-th Root of X(1:w949, 2:3.0 ("Exp. Voltage (V)")) -> (0:w936:dbl[])
                n256 = Multiply(x=w936, y=1000000.0 ("Exp. Voltage (V)")) -> (x*y=w946:dbl[])
              }
              frame "Charge" {
                n257 = case shown="\"Velocity\"" w979 {
                  tunnel: w978 -> [w983 w1014 _]
                  tunnel: [w983 w1014 w1018] -> w977
                  tunnel: w976 -> [w1007 w1013 _]
                  tunnel: [w1007 w1013 w1031] -> w975
                  tunnel: w974 -> [w1006 w1012 _]
                  tunnel: [w1006 w1012 w1030] -> w973
                  tunnel: w972 -> [w1005 w1011 _]
                  tunnel: [w1005 w1011 w1029] -> w971
                  tunnel: w970 -> [w988 w1010 w1016]
                  tunnel: [w988 w1010 w1016] -> w969
                  tunnel: w968 -> [_ w1009 w1017]
                  tunnel: [w984 w1009 w1017] -> w967
                  tunnel: w966 -> [_ w1008 w1019]
                  tunnel: [w985 w1008 w1019] -> w965
                  tunnel: w964 -> [w987 _ w1021]
                  tunnel: w963 -> [w986 _ _]
                  frame "Velocity" {
                    n258 = Multiply(x=1e-15 ("Exp. Voltage (V)"), y=w988) -> (x*y=w993:dbl[])
                    n259 = Multiply(x=w993, y=w987) -> (x*y=w998:dbl[])
                    n260 = Multiply(x=w983, y=1000.0 ("Exp. Voltage (V)")) -> (x*y=w990:dbl[])
                    n261 = Reverse 1D Array(array=w990) -> (reversed array=w980:dbl[])
                    n262 = Square(x=w980) -> (x^2=w995:dbl[])
                    n263 = Multiply(x=w998, y=2.0 ("Exp. Voltage (V)")) -> (x*y=w996:dbl[])
                    n264 = Divide(x=w996, y=w995) -> (x/y=w984:dbl[])
                    n265 = Multiply(x=w984, y=3.0 ("Exp. Voltage (V)")) -> (x*y=w1003:dbl[])
                    n266 = Divide(x=w1003, y=4.0 ("Exp. Voltage (V)")) -> (x/y=w1001:dbl[])
                    n267 = Divide(x=w1001, y=3.141592653589793) -> (x/y=w999:dbl[])
                    n268 = Divide(x=w999, y=w986) -> (x/y=w994:dbl[])
                    n269 = Y-th Root of X(1:w994, 2:3.0 ("Exp. Voltage (V)")) -> (0:w982:dbl[])
                    n270 = Multiply(x=w982, y=1000000.0 ("Exp. Voltage (V)")) -> (x*y=w985:dbl[])
                  }
                  frame "Charge" {
                  }
                  frame "Mass" {
                    w1038 = 99.989
                    w1036 = 1000000.0 ("y")
                    n271 = Multiply(x=w1016, y=1e-15 ("x")) -> (x*y=w1027:dbl[])
                    n272 = Reverse 1D Array(array=w1017) -> (reversed array=w1015:dbl[])
                    n273 = Multiply(x=w1027, y=w1021) -> (x*y=w1026:dbl[])
                    n274 = Divide(x=w1026, y=w1015) -> (x/y=w1025:dbl[])
                    n275 = Multiply(x=w1025, y=2.0 ("x")) -> (x*y=w1023:dbl[])
                    n276 = Square Root(x=w1023) -> (sqrt(x)=w1020:dbl[])
                    n277 = Index Array(array=w1020) -> (element #1=w1049:dbl, element #2=w1050:dbl)  [unwired: 2 in]
                    n278 = Divide(x=0.6, y=w1049) -> (x/y=w1034:dbl)
                    n279 = Divide(x=0.6, y=w1050) -> (x/y=w1035:dbl)
                    n280 = Subtract(x=w1034, y=w1035) -> (x-y=w1037:dbl)
                    n281 = Multiply(x=w1035, y=w1036) -> (x*y=w1044:dbl)
                    n282 = Multiply(x=w1037, y=w1036) -> (x*y=w1043:dbl)
                    n283 = Less?(x=w1044, y=w1038) -> (x < y?=w1039:bool)
                    n284 = Less?(x=w1043, y=w1038) -> (x < y?=w1040:bool)
                    n285 = Divide(x=w1020, y=1000.0 ("x")) -> (x/y=w1018:dbl[])
                    n286 = And(x=w1039, y=w1040) -> (x .and. y?=w1046:bool)
                    n287 = Select(t=u16 0 ("Multiplier"), s=w1046, f=u16 1 ("Multiplier")) -> (s? t:f=w1029:u16)
                    n288 = Select(t=10.0, s=w1046, f=1.0) -> (s? t:f=w1045:dbl)
                    n289 = Multiply(x=w1043, y=w1045) -> (x*y=w1031:dbl)
                    n290 = Multiply(x=w1044, y=w1045) -> (x*y=w1030:dbl)
                  }
                }
              }
              frame "Mass" {
                w1074 = 99.989
                w1072 = 1000000.0 ("y")
                n291 = Multiply(x=w1064, y=1e-15 ("x")) -> (x*y=w1062:dbl[])
                n292 = Multiply(x=w1062, y=w1061) -> (x*y=w1060:dbl[])
                n293 = Reverse 1D Array(array=w1059) -> (reversed array=w1051:dbl[])
                n294 = Divide(x=w1060, y=w1051) -> (x/y=w1058:dbl[])
                n295 = Multiply(x=w1058, y=2.0 ("x")) -> (x*y=w1056:dbl[])
                n296 = Square Root(x=w1056) -> (sqrt(x)=w1053:dbl[])
                n297 = Index Array(array=w1053) -> (element #1=w1085:dbl, element #2=w1086:dbl)  [unwired: 2 in]
                n298 = Divide(x=0.6, y=w1085) -> (x/y=w1070:dbl)
                n299 = Divide(x=0.6, y=w1086) -> (x/y=w1071:dbl)
                n300 = Subtract(x=w1070, y=w1071) -> (x-y=w1073:dbl)
                n301 = Multiply(x=w1071, y=w1072) -> (x*y=w1080:dbl)
                n302 = Multiply(x=w1073, y=w1072) -> (x*y=w1079:dbl)
                n303 = Divide(x=w1053, y=1000.0 ("x")) -> (x/y=w1054:dbl[])
                n304 = Less?(x=w1080, y=w1074) -> (x < y?=w1075:bool)
                n305 = Less?(x=w1079, y=w1074) -> (x < y?=w1076:bool)
                n306 = local write "Variable 2"(enum32{"Velocity", "Charge", "Mass"}."Charge" ("Variable 2")) -> ()
                n307 = And(x=w1075, y=w1076) -> (x .and. y?=w1082:bool)
                n308 = Select(t=u16 0 ("Multiplier"), s=w1082, f=u16 1 ("Multiplier")) -> (s? t:f=w1065:u16)
                n309 = Select(t=10.0, s=w1082, f=1.0) -> (s? t:f=w1081:dbl)
                n310 = Multiply(x=w1079, y=w1081) -> (x*y=w1067:dbl)
                n311 = Multiply(x=w1080, y=w1081) -> (x*y=w1066:dbl)
              }
            }
            n312 = Index Array(array=w911) -> (element #1=w912:dbl, element #2=w905:dbl)  [unwired: 2 in]
            n313 = Index Array(array=w910) -> (element #1=w907:dbl, element #2=w906:dbl)  [unwired: 2 in]
            n314 = Index Array(array=w908) -> (element #1=w902:dbl, element #2=w901:dbl)  [unwired: 2 in]
            n315 = Index Array(array=w909) -> (element #1=w904:dbl, element #2=w903:dbl)  [unwired: 2 in]
            n316 = Bundle By Name(cluster=w932, "Low speed (km/s)"=w912, "High speed (km/s)"=w905, "Window (Delta-T)"=w915, "Lower Cutoff"=w914, "Multiplier"=w913, "Low Charge (fC)"=w907, "High Charge (fC)"=w906, "Low Mass (kg)"=w904, "High Mass (kg)"=w903, "Low Radius (µm)"=w902, "High Radius (µm)"=w901, "Exp. Voltage (MV)"=w898) -> (w933:T1)
            n317 = local write "PSU Calc"(w933) -> ()
          }
          event Value Change {
            n318 = event-data() -> ()  [unwired: 1 in, 5 out]
            n319 = local read "PSU Calc"() -> (w1125:T1)
            n320 = Unbundle By Name(w1125) -> ("Low speed (km/s)"=w1124:dbl, "High speed (km/s)"=w1123:dbl, "Window (Delta-T)"=w1111:dbl, "Lower Cutoff"=w1110:dbl, "Multiplier"=w1109:u16, "Low Charge (fC)"=w1121:dbl, "High Charge (fC)"=w1120:dbl, "Low Mass (kg)"=w1119:dbl, "High Mass (kg)"=w1118:dbl, "Low Radius (µm)"=w1117:dbl, "High Radius (µm)"=w1116:dbl, "Exp. Voltage (MV)"=w1090:dbl)
            n321 = Build Array(w1117, w1116) -> (w1113:dbl[])
            n322 = Build Array(w1124, w1123) -> (w1122:dbl[])
            n323 = Build Array(w1121, w1120) -> (w1115:dbl[])
            n324 = Build Array(w1119, w1118) -> (w1114:dbl[])
            n325 = Multiply(x=w1090, y=1000000.0) -> (x*y=w1089:dbl)
            n326 = case shown="\"Mass\"" w1092 {
              tunnel: w1122 -> [w1143 w1229 w1295]
              tunnel: w1115 -> [w1142 w1228 w1294]
              tunnel: w1114 -> [w1141 w1227 w1293]
              tunnel: w1113 -> [w1140 w1226 w1292]
              tunnel: w1089 -> [w1139 w1225 w1291]
              tunnel: w1112 -> [w1138 w1224 w1290]
              tunnel: w1111 -> [w1137 w1223 w1289]
              tunnel: w1110 -> [w1136 w1222 w1288]
              tunnel: w1109 -> [w1135 w1221 w1287]
              tunnel: [w1134 w1220 w1286] -> w1108
              tunnel: [w1133 w1219 w1285] -> w1107
              tunnel: [w1132 w1218 w1284] -> w1106
              tunnel: [w1131 w1217 w1283] -> w1104
              tunnel: [w1130 w1216 w1282] -> w1103
              tunnel: [w1129 w1215 w1281] -> w1102
              tunnel: [w1128 w1214 w1280] -> w1101
              tunnel: w1093 -> [w1127 w1213 w1279]
              frame "Charge" {
                n327 = case shown="\"Mass\"" w1127 {
                  tunnel: w1143 -> [w1150 w1176 _]
                  tunnel: w1139 -> [w1163 _ w1186]
                  tunnel: w1142 -> [w1157 w1175 w1189]
                  tunnel: w1138 -> [w1162 _ _]
                  tunnel: w1141 -> [_ w1174 w1184]
                  tunnel: w1140 -> [_ w1173 w1212]
                  tunnel: [w1150 w1176 w1180] -> w1131
                  tunnel: [w1157 w1175 w1189] -> w1130
                  tunnel: [w1151 w1174 w1184] -> w1129
                  tunnel: [w1153 w1173 w1212] -> w1128
                  tunnel: w1137 -> [w1149 w1172 _]
                  tunnel: w1136 -> [w1148 w1171 _]
                  tunnel: w1135 -> [w1147 w1170 _]
                  tunnel: [w1149 w1172 w1192] -> w1134
                  tunnel: [w1148 w1171 w1191] -> w1133
                  tunnel: [w1147 w1170 w1190] -> w1132
                  frame "Velocity" {
                    n328 = Multiply(x=1e-15 ("Exp. Voltage (V)"), y=w1157) -> (x*y=w1155:dbl[])
                    n329 = Multiply(x=w1155, y=w1163) -> (x*y=w1161:dbl[])
                    n330 = Multiply(x=w1150, y=1000.0 ("Exp. Voltage (V)")) -> (x*y=w1146:dbl[])
                    n331 = Reverse 1D Array(array=w1146) -> (reversed array=w1144:dbl[])
                    n332 = Square(x=w1144) -> (x^2=w1158:dbl[])
                    n333 = Multiply(x=w1161, y=2.0 ("Exp. Voltage (V)")) -> (x*y=w1159:dbl[])
                    n334 = Divide(x=w1159, y=w1158) -> (x/y=w1151:dbl[])
                    n335 = Multiply(x=w1151, y=3.0 ("Exp. Voltage (V)")) -> (x*y=w1168:dbl[])
                    n336 = Divide(x=w1168, y=4.0 ("Exp. Voltage (V)")) -> (x/y=w1166:dbl[])
                    n337 = Divide(x=w1166, y=3.141592653589793) -> (x/y=w1164:dbl[])
                    n338 = Divide(x=w1164, y=w1162) -> (x/y=w1156:dbl[])
                    n339 = Multiply(x=w1156, y=1000000.0 ("Exp. Voltage (V)")) -> (x*y=w1153:dbl[])
                  }
                  frame "Charge" {
                  }
                  frame "Mass" {
                    w1199 = 99.989
                    w1197 = 1000000.0 ("y")
                    n340 = Multiply(x=w1189, y=1e-15 ("x")) -> (x*y=w1187:dbl[])
                    n341 = Multiply(x=w1187, y=w1186) -> (x*y=w1185:dbl[])
                    n342 = Reverse 1D Array(array=w1184) -> (reversed array=w1177:dbl[])
                    n343 = Divide(x=w1185, y=w1177) -> (x/y=w1183:dbl[])
                    n344 = Multiply(x=w1183, y=2.0 ("x")) -> (x*y=w1181:dbl[])
                    n345 = Square Root(x=w1181) -> (sqrt(x)=w1179:dbl[])
                    n346 = Index Array(array=w1179) -> (element #1=w1210:dbl, element #2=w1211:dbl)  [unwired: 2 in]
                    n347 = Divide(x=0.6, y=w1210) -> (x/y=w1195:dbl)
                    n348 = Divide(x=0.6, y=w1211) -> (x/y=w1196:dbl)
                    n349 = Subtract(x=w1195, y=w1196) -> (x-y=w1198:dbl)
                    n350 = Multiply(x=w1196, y=w1197) -> (x*y=w1205:dbl)
                    n351 = Multiply(x=w1198, y=w1197) -> (x*y=w1204:dbl)
                    n352 = Divide(x=w1179, y=1000.0 ("x")) -> (x/y=w1180:dbl[])
                    n353 = Less?(x=w1205, y=w1199) -> (x < y?=w1200:bool)
                    n354 = Less?(x=w1204, y=w1199) -> (x < y?=w1201:bool)
                    n355 = And(x=w1200, y=w1201) -> (x .and. y?=w1207:bool)
                    n356 = Select(t=u16 0 ("Multiplier"), s=w1207, f=u16 1 ("Multiplier")) -> (s? t:f=w1190:u16)
                    n357 = Select(t=10.0, s=w1207, f=1.0) -> (s? t:f=w1206:dbl)
                    n358 = Multiply(x=w1204, y=w1206) -> (x*y=w1192:dbl)
                    n359 = Multiply(x=w1205, y=w1206) -> (x*y=w1191:dbl)
                  }
                }
              }
              frame "Velocity" {
                n360 = case shown="\"Charge\"" w1213 {
                  tunnel: w1229 -> [w1236 w1243 w1268]
                  tunnel: w1225 -> [_ w1256 w1266]
                  tunnel: w1228 -> [w1235 w1250 _]
                  tunnel: w1224 -> [_ w1255 _]
                  tunnel: w1227 -> [w1234 _ w1267]
                  tunnel: w1226 -> [w1233 _ w1275]
                  tunnel: [w1236 w1243 w1268] -> w1217
                  tunnel: [w1235 w1250 w1265] -> w1216
                  tunnel: [w1234 w1244 w1267] -> w1215
                  tunnel: [w1233 w1246 w1275] -> w1214
                  tunnel: w1223 -> [w1232 w1242 w1278]
                  tunnel: w1222 -> [w1231 w1241 w1277]
                  tunnel: w1221 -> [w1230 w1240 w1276]
                  tunnel: [w1232 w1242 w1278] -> w1220
                  tunnel: [w1231 w1241 w1277] -> w1219
                  tunnel: [w1230 w1240 w1276] -> w1218
                  frame "Velocity" {
                  }
                  frame "Charge" {
                    n361 = Multiply(x=1e-15 ("Exp. Voltage (V)"), y=w1250) -> (x*y=w1248:dbl[])
                    n362 = Multiply(x=w1248, y=w1256) -> (x*y=w1254:dbl[])
                    n363 = Multiply(x=w1243, y=1000.0 ("Exp. Voltage (V)")) -> (x*y=w1239:dbl[])
                    n364 = Reverse 1D Array(array=w1239) -> (reversed array=w1237:dbl[])
                    n365 = Square(x=w1237) -> (x^2=w1251:dbl[])
                    n366 = Multiply(x=w1254, y=2.0 ("Exp. Voltage (V)")) -> (x*y=w1252:dbl[])
                    n367 = Divide(x=w1252, y=w1251) -> (x/y=w1244:dbl[])
                    n368 = Multiply(x=w1244, y=3.0 ("Exp. Voltage (V)")) -> (x*y=w1261:dbl[])
                    n369 = Divide(x=w1261, y=4.0 ("Exp. Voltage (V)")) -> (x/y=w1259:dbl[])
                    n370 = Divide(x=w1259, y=3.141592653589793) -> (x/y=w1257:dbl[])
                    n371 = Divide(x=w1257, y=w1255) -> (x/y=w1249:dbl[])
                    n372 = Multiply(x=w1249, y=1000000.0 ("Exp. Voltage (V)")) -> (x*y=w1246:dbl[])
                  }
                  frame "Mass" {
                    n373 = Divide(x=w1267, y=w1266) -> (x/y=w1274:dbl[])
                    n374 = Multiply(x=w1268, y=1000.0 ("Exp. Voltage (V)")) -> (x*y=w1264:dbl[])
                    n375 = Square(x=w1264) -> (x^2=w1271:dbl[])
                    n376 = Divide(x=w1274, y=2.0 ("Exp. Voltage (V)")) -> (x/y=w1272:dbl[])
                    n377 = Multiply(x=w1272, y=w1271) -> (x*y=w1270:dbl[])
                    n378 = Multiply(x=w1270, y=1000000000000000.0 ("Exp. Voltage (V)")) -> (x*y=w1265:dbl[])
                  }
                }
              }
              frame "Mass" {
                n379 = case shown="\"Velocity\"" w1279 {
                  tunnel: w1295 -> [w1301 _ w1354]
                  tunnel: w1291 -> [w1305 w1318 _]
                  tunnel: w1294 -> [_ w1319 w1353]
                  tunnel: w1290 -> [_ _ _]
                  tunnel: w1293 -> [w1302 w1322 w1352]
                  tunnel: w1292 -> [w1303 w1321 w1351]
                  tunnel: [w1301 w1314 w1354] -> w1283
                  tunnel: [w1297 w1319 w1353] -> w1282
                  tunnel: [w1302 w1322 w1352] -> w1281
                  tunnel: [w1303 w1321 w1351] -> w1280
                  tunnel: w1289 -> [w1300 _ w1350]
                  tunnel: w1288 -> [w1299 _ w1349]
                  tunnel: w1287 -> [w1298 _ w1348]
                  tunnel: [w1300 w1315 w1350] -> w1286
                  tunnel: [w1299 w1316 w1349] -> w1285
                  tunnel: [w1298 w1317 w1348] -> w1284
                  frame "Velocity" {
                    n380 = Multiply(x=w1301, y=1000.0 ("Lower Cutoff")) -> (x*y=w1308:dbl[])
                    n381 = Divide(x=w1302, y=2.0 ("Lower Cutoff")) -> (x/y=w1309:dbl[])
                    n382 = Square(x=w1308) -> (x^2=w1310:dbl[])
                    n383 = Multiply(x=w1310, y=w1309) -> (x*y=w1306:dbl[])
                    n384 = Divide(x=w1306, y=w1305) -> (x/y=w1304:dbl[])
                    n385 = Multiply(x=w1304, y=1000000000000000.0 ("Lower Cutoff")) -> (x*y=w1297:dbl[])
                  }
                  frame "Charge" {
                    w1335 = 99.989
                    w1333 = 1000000.0 ("y")
                    n386 = Multiply(x=w1319, y=1e-15 ("x")) -> (x*y=w1327:dbl[])
                    n387 = Multiply(x=w1327, y=w1318) -> (x*y=w1326:dbl[])
                    n388 = Reverse 1D Array(array=w1322) -> (reversed array=w1312:dbl[])
                    n389 = Divide(x=w1326, y=w1312) -> (x/y=w1325:dbl[])
                    n390 = Multiply(x=w1325, y=2.0 ("x")) -> (x*y=w1323:dbl[])
                    n391 = Square Root(x=w1323) -> (sqrt(x)=w1320:dbl[])
                    n392 = Index Array(array=w1320) -> (element #1=w1346:dbl, element #2=w1347:dbl)  [unwired: 2 in]
                    n393 = Divide(x=0.6, y=w1346) -> (x/y=w1331:dbl)
                    n394 = Divide(x=0.6, y=w1347) -> (x/y=w1332:dbl)
                    n395 = Subtract(x=w1331, y=w1332) -> (x-y=w1334:dbl)
                    n396 = Multiply(x=w1332, y=w1333) -> (x*y=w1341:dbl)
                    n397 = Multiply(x=w1334, y=w1333) -> (x*y=w1340:dbl)
                    n398 = Less?(x=w1341, y=w1335) -> (x < y?=w1336:bool)
                    n399 = Less?(x=w1340, y=w1335) -> (x < y?=w1337:bool)
                    n400 = Divide(x=w1320, y=1000.0 ("x")) -> (x/y=w1314:dbl[])
                    n401 = And(x=w1336, y=w1337) -> (x .and. y?=w1343:bool)
                    n402 = Select(t=u16 0 ("Multiplier"), s=w1343, f=u16 1 ("Multiplier")) -> (s? t:f=w1317:u16)
                    n403 = Select(t=10.0, s=w1343, f=1.0) -> (s? t:f=w1342:dbl)
                    n404 = Multiply(x=w1340, y=w1342) -> (x*y=w1315:dbl)
                    n405 = Multiply(x=w1341, y=w1342) -> (x*y=w1316:dbl)
                  }
                  frame "Mass" {
                  }
                }
              }
            }
            n406 = Index Array(array=w1104) -> (element #1=w1105:dbl, element #2=w1098:dbl)  [unwired: 2 in]
            n407 = Index Array(array=w1103) -> (element #1=w1100:dbl, element #2=w1099:dbl)  [unwired: 2 in]
            n408 = Index Array(array=w1101) -> (element #1=w1095:dbl, element #2=w1094:dbl)  [unwired: 2 in]
            n409 = Index Array(array=w1102) -> (element #1=w1097:dbl, element #2=w1096:dbl)  [unwired: 2 in]
            n410 = Bundle By Name(cluster=w1125, "Low speed (km/s)"=w1105, "High speed (km/s)"=w1098, "Window (Delta-T)"=w1108, "Lower Cutoff"=w1107, "Multiplier"=w1106, "Low Charge (fC)"=w1100, "High Charge (fC)"=w1099, "Low Mass (kg)"=w1097, "High Mass (kg)"=w1096, "Low Radius (µm)"=w1095, "High Radius (µm)"=w1094, "Exp. Voltage (MV)"=w1090) -> (w1126:T1)
            n411 = local write "PSU Calc"(w1126) -> ()
          }
          event "Variable 1": Value Change {
            n412 = event-data() -> ("OldVal"=w1360:enum32{"Velocity", "Charge", "Mass"}, "NewVal"=w1362:enum32{"Velocity", "Charge", "Mass"})  [unwired: 1 in, 3 out]
            n413 = property on="Variable 2" class="RadioBtnsControl (strict)"(error in=w1363) -> (error out=w1364:errorcluster, "Controls[]"=w1369:refnum<vi>[])  [unwired: 1 in, 1 out]
            n414 = Index Array(array=w1369, index=w1360) -> (element=w1368:refnum<vi>)
            n415 = Index Array(array=w1369, index=w1362) -> (element=w1367:refnum<vi>)
            n416 = property class="Ctl"(reference=w1368, error in=w1364, "DisabledEnum"=T2."Enabled" ("Disabled")) -> (error out=w1357:errorcluster)  [unwired: 1 out]
            n417 = property class="Ctl"(reference=w1367, error in=w1364, "DisabledEnum"=T2."Disabled and Grayed Out" ("Disabled")) -> (error out=w1356:errorcluster)  [unwired: 1 out]
            n418 = Equal?(x=w1362, y=w1359) -> (x = y?=w1361:bool)
            n419 = Select(t=w1360, s=w1361, f=w1359) -> (s? t:f=w1358:enum32{"Velocity", "Charge", "Mass"})
            n420 = Merge Errors(w1357, w1356) -> (w1355:errorcluster)
            n421 = local write "Variable 2"(w1358) -> ()
          }
          event Value Change {
            n422 = event-data() -> ()  [unwired: 1 in, 5 out]
            n423 = local read "PSU Calc"() -> (w1414:T1)
            n424 = Unbundle By Name(w1414) -> ("Low speed (km/s)"=w1413:dbl, "High speed (km/s)"=w1412:dbl, "Window (Delta-T)"=w1405:dbl, "Lower Cutoff"=w1404:dbl, "Multiplier"=w1403:u16, "Low Charge (fC)"=w1410:dbl, "High Charge (fC)"=w1409:dbl, "Low Mass (kg)"=w1408:dbl, "High Mass (kg)"=w1407:dbl, "Exp. Voltage (MV)"=w1373:dbl)  [unwired: 2 out]
            n425 = Build Array(w1413, w1412) -> (w1411:dbl[])
            n426 = Build Array(w1410, w1409) -> (w1406:dbl[])
            n427 = Build Array(w1408, w1407) -> (w1387:dbl[])
            n428 = Multiply(x=1000000.0, y=w1373) -> (x*y=w1372:dbl)
            n429 = Multiply(x=w1387, y=3.0 ("x")) -> (x*y=w1385:dbl[])
            n430 = Divide(x=w1385, y=4.0 ("x")) -> (x/y=w1383:dbl[])
            n431 = case shown="\"Velocity\"" w1388 {
              tunnel: w1411 -> [w1425 _ w1480]
              tunnel: w1372 -> [w1419 w1442 w1468]
              tunnel: w1406 -> [_ w1445 w1472]
              tunnel: w1387 -> [w1427 w1440 w1469]
              tunnel: [w1425 w1435 w1479] -> w1398
              tunnel: [w1417 w1445 w1471] -> w1397
              tunnel: [w1427 w1440 w1470] -> w1396
              tunnel: w1405 -> [w1431 _ w1478]
              tunnel: w1404 -> [w1430 _ w1476]
              tunnel: w1403 -> [w1429 _ w1474]
              tunnel: [w1431 w1448 w1477] -> w1402
              tunnel: [w1430 w1447 w1475] -> w1401
              tunnel: [w1429 w1446 w1473] -> w1400
              tunnel: w1370 -> [_ _ w1481]
              frame "Velocity" {
                n432 = Multiply(x=w1425, y=1000.0 ("Lower Cutoff")) -> (x*y=w1422:dbl[])
                n433 = Divide(x=w1427, y=2.0 ("Lower Cutoff")) -> (x/y=w1423:dbl[])
                n434 = Square(x=w1422) -> (x^2=w1424:dbl[])
                n435 = Multiply(x=w1424, y=w1423) -> (x*y=w1420:dbl[])
                n436 = Divide(x=w1420, y=w1419) -> (x/y=w1418:dbl[])
                n437 = Multiply(x=1000000000000000.0 ("Lower Cutoff"), y=w1418) -> (x*y=w1417:dbl[])
                n438 = local write "Variable 2"(enum32{"Velocity", "Charge", "Mass"}."Mass" ("Variable 2")) -> ()
              }
              frame "Charge" {
                w1455 = 99.989
                w1453 = 1000000.0 ("y")
                n439 = Multiply(x=w1445, y=1e-15 ("x")) -> (x*y=w1443:dbl[])
                n440 = Multiply(x=w1443, y=w1442) -> (x*y=w1441:dbl[])
                n441 = Reverse 1D Array(array=w1440) -> (reversed array=w1432:dbl[])
                n442 = Divide(x=w1441, y=w1432) -> (x/y=w1439:dbl[])
                n443 = Multiply(x=w1439, y=2.0 ("x")) -> (x*y=w1437:dbl[])
                n444 = Square Root(x=w1437) -> (sqrt(x)=w1434:dbl[])
                n445 = Index Array(array=w1434) -> (element #1=w1466:dbl, element #2=w1467:dbl)  [unwired: 2 in]
                n446 = Divide(x=0.6, y=w1466) -> (x/y=w1451:dbl)
                n447 = Divide(x=0.6, y=w1467) -> (x/y=w1452:dbl)
                n448 = Subtract(x=w1451, y=w1452) -> (x-y=w1454:dbl)
                n449 = Multiply(x=w1452, y=w1453) -> (x*y=w1461:dbl)
                n450 = Multiply(x=w1454, y=w1453) -> (x*y=w1460:dbl)
                n451 = Divide(x=w1434, y=1000.0) -> (x/y=w1435:dbl[])
                n452 = Less?(x=w1461, y=w1455) -> (x < y?=w1456:bool)
                n453 = Less?(x=w1460, y=w1455) -> (x < y?=w1457:bool)
                n454 = local write "Variable 2"(enum32{"Velocity", "Charge", "Mass"}."Mass" ("Variable 2")) -> ()
                n455 = And(x=w1456, y=w1457) -> (x .and. y?=w1463:bool)
                n456 = Select(t=u16 0 ("Multiplier"), s=w1463, f=u16 1 ("Multiplier")) -> (s? t:f=w1446:u16)
                n457 = Select(t=10.0, s=w1463, f=1.0) -> (s? t:f=w1462:dbl)
                n458 = Multiply(x=w1460, y=w1462) -> (x*y=w1448:dbl)
                n459 = Multiply(x=w1461, y=w1462) -> (x*y=w1447:dbl)
              }
              frame "Mass" {
                n460 = case shown="\"Charge\"" w1481 {
                  tunnel: w1480 -> [w1484 _ w1537]
                  tunnel: [w1484 w1498 w1537] -> w1479
                  tunnel: w1478 -> [w1488 _ w1536]
                  tunnel: [w1488 w1512 w1536] -> w1477
                  tunnel: w1476 -> [w1487 _ w1535]
                  tunnel: [w1487 w1511 w1535] -> w1475
                  tunnel: w1474 -> [w1486 _ w1534]
                  tunnel: [w1486 w1510 w1534] -> w1473
                  tunnel: w1472 -> [_ w1501 w1533]
                  tunnel: [w1489 w1501 w1533] -> w1471
                  tunnel: [w1482 w1499 w1532] -> w1470
                  tunnel: w1469 -> [w1482 w1499 w1532]
                  tunnel: w1468 -> [w1490 w1500 _]
                  frame "Velocity" {
                    n461 = Multiply(x=w1484, y=1000.0 ("x")) -> (x*y=w1485:dbl[])
                    n462 = Square(x=w1485) -> (x^2=w1494:dbl[])
                    n463 = Divide(x=w1482, y=2.0 ("x")) -> (x/y=w1495:dbl[])
                    n464 = Multiply(x=w1494, y=w1495) -> (x*y=w1493:dbl[])
                    n465 = Divide(x=w1493, y=w1490) -> (x/y=w1492:dbl[])
                    n466 = Multiply(x=1000000000000000.0, y=w1492) -> (x*y=w1489:dbl[])
                  }
                  frame "Charge" {
                    w1525 = 99.989
                    w1527 = 1000000.0 ("y")
                    n467 = Multiply(x=w1501, y=1e-15 ("x")) -> (x*y=w1508:dbl[])
                    n468 = Multiply(x=w1508, y=w1500) -> (x*y=w1507:dbl[])
                    n469 = Reverse 1D Array(array=w1499) -> (reversed array=w1497:dbl[])
                    n470 = Divide(x=w1507, y=w1497) -> (x/y=w1506:dbl[])
                    n471 = Multiply(x=w1506, y=2.0 ("x")) -> (x*y=w1504:dbl[])
                    n472 = Square Root(x=w1504) -> (sqrt(x)=w1502:dbl[])
                    n473 = Index Array(array=w1502) -> (element #1=w1514:dbl, element #2=w1513:dbl)  [unwired: 2 in]
                    n474 = Divide(x=0.6, y=w1514) -> (x/y=w1529:dbl)
                    n475 = Divide(x=0.6, y=w1513) -> (x/y=w1528:dbl)
                    n476 = Subtract(x=w1529, y=w1528) -> (x-y=w1526:dbl)
                    n477 = Multiply(x=w1528, y=w1527) -> (x*y=w1519:dbl)
                    n478 = Multiply(x=w1526, y=w1527) -> (x*y=w1520:dbl)
                    n479 = Less?(x=w1519, y=w1525) -> (x < y?=w1524:bool)
                    n480 = Less?(x=w1520, y=w1525) -> (x < y?=w1523:bool)
                    n481 = Divide(x=w1502, y=1000.0 ("x")) -> (x/y=w1498:dbl[])
                    n482 = And(x=w1524, y=w1523) -> (x .and. y?=w1517:bool)
                    n483 = Select(t=u16 0 ("Multiplier"), s=w1517, f=u16 1 ("Multiplier")) -> (s? t:f=w1510:u16)
                    n484 = Select(t=10.0, s=w1517, f=1.0) -> (s? t:f=w1518:dbl)
                    n485 = Multiply(x=w1520, y=w1518) -> (x*y=w1512:dbl)
                    n486 = Multiply(x=w1519, y=w1518) -> (x*y=w1511:dbl)
                  }
                  frame "Mass" {
                  }
                }
              }
            }
            n487 = Divide(x=w1383, y=3.141592653589793) -> (x/y=w1381:dbl[])
            n488 = Divide(x=w1381, y=w1380) -> (x/y=w1379:dbl[])
            n489 = Y-th Root of X(1:w1379, 2:3.0 ("x")) -> (0:w1377:dbl[])
            n490 = Multiply(x=w1377, y=1000000.0 ("x")) -> (x*y=w1375:dbl[])
            n491 = Index Array(array=w1398) -> (element #1=w1399:dbl, element #2=w1393:dbl)  [unwired: 2 in]
            n492 = Index Array(array=w1397) -> (element #1=w1395:dbl, element #2=w1394:dbl)  [unwired: 2 in]
            n493 = Index Array(array=w1375) -> (element #1=w1390:dbl, element #2=w1389:dbl)  [unwired: 2 in]
            n494 = Index Array(array=w1396) -> (element #1=w1392:dbl, element #2=w1391:dbl)  [unwired: 2 in]
            n495 = Bundle By Name(cluster=w1414, "Low speed (km/s)"=w1399, "High speed (km/s)"=w1393, "Window (Delta-T)"=w1402, "Lower Cutoff"=w1401, "Multiplier"=w1400, "Low Charge (fC)"=w1395, "High Charge (fC)"=w1394, "Low Mass (kg)"=w1392, "High Mass (kg)"=w1391, "Low Radius (µm)"=w1390, "High Radius (µm)"=w1389, "Exp. Voltage (MV)"=w1373) -> (w1415:T1)
            n496 = local write "PSU Calc"(w1415) -> ()
            "Dust Density\n(kg/m^3)" <- w1380
          }
          event Value Change {
            n497 = event-data() -> ()  [unwired: 1 in, 5 out]
            n498 = local read "PSU Calc"() -> (w1582:T1)
            n499 = Unbundle By Name(w1582) -> ("Low speed (km/s)"=w1581:dbl, "High speed (km/s)"=w1580:dbl, "Window (Delta-T)"=w1575:dbl, "Lower Cutoff"=w1574:dbl, "Multiplier"=w1573:u16, "Low Charge (fC)"=w1578:dbl, "High Charge (fC)"=w1577:dbl, "Low Radius (µm)"=w1550:dbl, "High Radius (µm)"=w1549:dbl, "Exp. Voltage (MV)"=w1541:dbl)  [unwired: 2 out]
            n500 = Multiply(x=w1541, y=1000000.0) -> (x*y=w1540:dbl)
            n501 = Build Array(w1581, w1580) -> (w1579:dbl[])
            n502 = Build Array(w1578, w1577) -> (w1576:dbl[])
            n503 = Build Array(w1550, w1549) -> (w1546:dbl[])
            n504 = Divide(x=w1546, y=1000000.0 ("x")) -> (x/y=w1544:dbl[])
            n505 = Power Of X(1:w1544, 2:3.0 ("x")) -> (0:w1547:dbl[])
            n506 = Divide(x=w1547, y=3.0 ("x")) -> (x/y=w1556:dbl[])
            n507 = Multiply(x=w1556, y=4.0 ("x")) -> (x*y=w1554:dbl[])
            n508 = Multiply(x=w1554, y=3.141592653589793) -> (x*y=w1552:dbl[])
            n509 = Multiply(x=w1552, y=w1551) -> (x*y=w1548:dbl[])
            n510 = case shown="\"Mass\"" w1558 {
              tunnel: w1579 -> [w1593 _ w1647]
              tunnel: w1540 -> [w1587 w1608 w1637]
              tunnel: w1576 -> [_ w1611 w1639]
              tunnel: w1548 -> [w1595 w1606 w1636]
              tunnel: [w1593 w1602 w1646] -> w1568
              tunnel: [w1585 w1611 w1638] -> w1567
              tunnel: [w1595 w1606 w1635] -> w1566
              tunnel: w1575 -> [w1599 _ w1645]
              tunnel: w1574 -> [w1598 _ w1643]
              tunnel: w1573 -> [w1597 _ w1641]
              tunnel: [w1599 w1614 w1644] -> w1572
              tunnel: [w1598 w1613 w1642] -> w1571
              tunnel: [w1597 w1612 w1640] -> w1570
              tunnel: w1538 -> [_ _ w1634]
              frame "Velocity" {
                n511 = Multiply(x=w1593, y=1000.0 ("Lower Cutoff")) -> (x*y=w1590:dbl[])
                n512 = Divide(x=w1595, y=2.0 ("Lower Cutoff")) -> (x/y=w1591:dbl[])
                n513 = Square(x=w1590) -> (x^2=w1592:dbl[])
                n514 = Multiply(x=w1592, y=w1591) -> (x*y=w1588:dbl[])
                n515 = Divide(x=w1588, y=w1587) -> (x/y=w1586:dbl[])
                n516 = Multiply(x=1000000000000000.0 ("Lower Cutoff"), y=w1586) -> (x*y=w1585:dbl[])
                n517 = local write "Variable 2"(enum32{"Velocity", "Charge", "Mass"}."Mass" ("Variable 2")) -> ()
              }
              frame "Charge" {
                w1621 = 99.989
                w1619 = 1000000.0 ("y")
                n518 = Multiply(x=w1611, y=1e-15 ("x")) -> (x*y=w1609:dbl[])
                n519 = Multiply(x=w1609, y=w1608) -> (x*y=w1607:dbl[])
                n520 = Reverse 1D Array(array=w1606) -> (reversed array=w1600:dbl[])
                n521 = Divide(x=w1607, y=w1600) -> (x/y=w1605:dbl[])
                n522 = Multiply(x=w1605, y=2.0 ("x")) -> (x*y=w1603:dbl[])
                n523 = Square Root(x=w1603) -> (sqrt(x)=w1602:dbl[])
                n524 = Index Array(array=w1602) -> (element #1=w1632:dbl, element #2=w1633:dbl)  [unwired: 2 in]
                n525 = Divide(x=0.6, y=w1632) -> (x/y=w1617:dbl)
                n526 = Divide(x=0.6, y=w1633) -> (x/y=w1618:dbl)
                n527 = Subtract(x=w1617, y=w1618) -> (x-y=w1620:dbl)
                n528 = Multiply(x=w1618, y=w1619) -> (x*y=w1627:dbl)
                n529 = Multiply(x=w1620, y=w1619) -> (x*y=w1626:dbl)
                n530 = Less?(x=w1627, y=w1621) -> (x < y?=w1622:bool)
                n531 = Less?(x=w1626, y=w1621) -> (x < y?=w1623:bool)
                n532 = local write "Variable 2"(enum32{"Velocity", "Charge", "Mass"}."Mass" ("Variable 2")) -> ()
                n533 = And(x=w1622, y=w1623) -> (x .and. y?=w1629:bool)
                n534 = Select(t=u16 0 ("Multiplier"), s=w1629, f=u16 1 ("Multiplier")) -> (s? t:f=w1612:u16)
                n535 = Select(t=10.0, s=w1629, f=1.0) -> (s? t:f=w1628:dbl)
                n536 = Multiply(x=w1626, y=w1628) -> (x*y=w1614:dbl)
                n537 = Multiply(x=w1627, y=w1628) -> (x*y=w1613:dbl)
              }
              frame "Mass" {
                n538 = case shown="\"Velocity\"" w1634 {
                  tunnel: w1647 -> [w1650 _ w1703]
                  tunnel: [w1650 w1664 w1703] -> w1646
                  tunnel: w1645 -> [w1654 _ w1702]
                  tunnel: [w1654 w1678 w1702] -> w1644
                  tunnel: w1643 -> [w1653 _ w1701]
                  tunnel: [w1653 w1677 w1701] -> w1642
                  tunnel: w1641 -> [w1652 _ w1700]
                  tunnel: [w1652 w1676 w1700] -> w1640
                  tunnel: w1639 -> [_ w1667 w1699]
                  tunnel: [w1655 w1667 w1699] -> w1638
                  tunnel: [w1648 w1665 w1698] -> w1635
                  tunnel: w1636 -> [w1648 w1665 w1698]
                  tunnel: w1637 -> [w1656 w1666 _]
                  frame "Velocity" {
                    n539 = Multiply(x=w1650, y=1000.0 ("x")) -> (x*y=w1651:dbl[])
                    n540 = Square(x=w1651) -> (x^2=w1660:dbl[])
                    n541 = Divide(x=w1648, y=2.0 ("x")) -> (x/y=w1661:dbl[])
                    n542 = Multiply(x=w1660, y=w1661) -> (x*y=w1659:dbl[])
                    n543 = Divide(x=w1659, y=w1656) -> (x/y=w1658:dbl[])
                    n544 = Multiply(x=1000000000000000.0, y=w1658) -> (x*y=w1655:dbl[])
                  }
                  frame "Charge" {
                    w1691 = 99.989
                    w1693 = 1000000.0 ("y")
                    n545 = Multiply(x=w1667, y=1e-15 ("x")) -> (x*y=w1674:dbl[])
                    n546 = Multiply(x=w1674, y=w1666) -> (x*y=w1673:dbl[])
                    n547 = Reverse 1D Array(array=w1665) -> (reversed array=w1663:dbl[])
                    n548 = Divide(x=w1673, y=w1663) -> (x/y=w1672:dbl[])
                    n549 = Multiply(x=w1672, y=2.0 ("x")) -> (x*y=w1670:dbl[])
                    n550 = Square Root(x=w1670) -> (sqrt(x)=w1668:dbl[])
                    n551 = Index Array(array=w1668) -> (element #1=w1680:dbl, element #2=w1679:dbl)  [unwired: 2 in]
                    n552 = Divide(x=0.6, y=w1680) -> (x/y=w1695:dbl)
                    n553 = Divide(x=0.6, y=w1679) -> (x/y=w1694:dbl)
                    n554 = Subtract(x=w1695, y=w1694) -> (x-y=w1692:dbl)
                    n555 = Multiply(x=w1694, y=w1693) -> (x*y=w1685:dbl)
                    n556 = Multiply(x=w1692, y=w1693) -> (x*y=w1686:dbl)
                    n557 = Less?(x=w1685, y=w1691) -> (x < y?=w1690:bool)
                    n558 = Less?(x=w1686, y=w1691) -> (x < y?=w1689:bool)
                    n559 = Divide(x=w1668, y=1000.0 ("x")) -> (x/y=w1664:dbl[])
                    n560 = And(x=w1690, y=w1689) -> (x .and. y?=w1683:bool)
                    n561 = Select(t=u16 0 ("Multiplier"), s=w1683, f=u16 1 ("Multiplier")) -> (s? t:f=w1676:u16)
                    n562 = Select(t=10.0, s=w1683, f=1.0) -> (s? t:f=w1684:dbl)
                    n563 = Multiply(x=w1686, y=w1684) -> (x*y=w1678:dbl)
                    n564 = Multiply(x=w1685, y=w1684) -> (x*y=w1677:dbl)
                  }
                  frame "Mass" {
                  }
                }
              }
            }
            n565 = Index Array(array=w1568) -> (element #1=w1569:dbl, element #2=w1563:dbl)  [unwired: 2 in]
            n566 = Index Array(array=w1567) -> (element #1=w1565:dbl, element #2=w1564:dbl)  [unwired: 2 in]
            n567 = Index Array(array=w1546) -> (element #1=w1560:dbl, element #2=w1559:dbl)  [unwired: 2 in]
            n568 = Index Array(array=w1566) -> (element #1=w1562:dbl, element #2=w1561:dbl)  [unwired: 2 in]
            n569 = Bundle By Name(cluster=w1582, "Low speed (km/s)"=w1569, "High speed (km/s)"=w1563, "Window (Delta-T)"=w1572, "Lower Cutoff"=w1571, "Multiplier"=w1570, "Low Charge (fC)"=w1565, "High Charge (fC)"=w1564, "Low Mass (kg)"=w1562, "High Mass (kg)"=w1561, "Low Radius (µm)"=w1560, "High Radius (µm)"=w1559, "Exp. Voltage (MV)"=w1541) -> (w1583:T1)
            n570 = local write "PSU Calc"(w1583) -> ()
          }
        }
        n571 = Or(x="PSU update", y="OK1") -> (x .or. y?=w541:bool)
        n572 = Or(x="Cancel", y=w541) -> (x .or. y?=w537:bool)
        n573 = Not(x=w539) -> (.not. x?=w538:bool)
        n574 = Compound Arithmetic op=OR(w538, w536, w537) -> (w535:bool)
        n575 = And(x="Cancel", y=w535) -> ()  [unwired: 1 out]
        n576 = flat-sequence {
          tunnel: [w545] -> w531
          tunnel: w530 -> [w545]
          tunnel: [w544] -> w529
          frame #0 {
            n577 = local read "PSU Calc"() -> (w544:T1)
          }
        }
        n578 = Wait Until Next ms Multiple(millisecond multiple=u32 50) -> ()  [unwired: 1 out]
      }
      "OK" <- w70
      "Cancel 2" <- w61
      n579 = case shown="False" w61 {
        tunnel: w60 -> [w116 w121]
        tunnel: [w105 w121] -> w59
        tunnel: w58 -> [w120 _]
        frame False {
          n580 = Get Date/Time In Seconds() -> (seconds since 1Jan1904=w114:timestamp)
          n581 = global write "PSU updated.vi" "PSU updated"(TRUE ("PSU updated")) -> ()
          n582 = Unbundle By Name(w120) -> ("Low speed (km/s)"=w118:dbl, "High speed (km/s)"=w117:dbl, "Low Charge (fC)"=w102:dbl, "High Charge (fC)"=w103:dbl, "High Mass (kg)"=w101:dbl, "Low Mass (kg)"=w100:dbl)
          n583 = local read "Variable 1"() -> (w99:enum32{"Velocity", "Charge", "Mass"})
          n584 = local read "Variable 2"() -> (w98:enum32{"Velocity", "Charge", "Mass"})
          n585 = call "timestamp_conversion.vi"("error in (no error)"=w116, "Time Stamp"=w114) -> ("error out"=w113:errorcluster, "Integer Time"=w115:i64)  [unwired: 7 in]
          n586 = Bundle By Name(cluster=T3 {"Integer Timestamp"=0.0, "Max Velocity"=0.0, "Min Velocity"=0.0, "Max Charge"=0.0, "Min Charge"=0.0, "Max Mass"=0.0, "Min Mass"=0.0, "Variable 1"=enum."Mass", "Variable 2"=enum."Mass"} ("PSU settings"), "Integer Timestamp"=w115, "Max Velocity"=w117, "Min Velocity"=w118, "Max Charge"=w103, "Min Charge"=w102, "Max Mass"=w101, "Min Mass"=w100, "Variable 1"=w99, "Variable 2"=w98) -> (w110:T3)
          n587 = call "connect in.vi"("error in (no error)"=w113) -> ("error out"=w108:errorcluster, "Database Connection"=w111:T4)  [unwired: 6 in, 1 out]
          n588 = call <vilib>:"DB Tools Insert Data.vi"("data"=w110, "error in (no error)"=w108, "table"="psu", "connection reference"=w111) -> ("error out"=w107:errorcluster, "connection reference out"=w109:T4)  [unwired: 6 in]
          n589 = call "connect out.vi"("error in (no error)"=w108, "connection reference"=w109) -> ("error out"=w106:errorcluster)  [unwired: 9 in]
          n590 = Merge Errors(w107, w106) -> (w105:errorcluster)
        }
        frame True {
        }
      }
      n591 = Not(x=w75) -> (.not. x?=w74:bool)
      n592 = property class="VI"(error in=w59, "Front Panel Window:Open"=w74) -> (error out=w68:errorcluster)  [unwired: 1 in, 1 out]
    }
    frame Error {
    }
  }
  "error out" <- w1
